vi "Martins HOT interface Mikrotron.vi"() -> ()   [LabVIEW 2012]
uses:
  Sub VIs/Trap cluster.ctl
  <vilib>/vision/Image Controls.llb/IMAQ Image.ctl
  Sub VIs/Get measurement coordinates.vi
  Sub VIs/Global variables.vi
  <vilib>/Utility/inputDevices.llb/closeKeyboard.vi
  <vilib>/Utility/inputDevices.llb/keyboardAcquire.vi
  <vilib>/Utility/file.llb/Write To Spreadsheet File (DBL).vi
  Sub VIs/Get trap pos.vi
  <vilib>/Analysis/coordinate.llb/2D Cartesian Coordinate Shift.vi
  <vilib>/Analysis/coordinate.llb/2D Cartesian Coordinate Shift (Array).vi
  <vilib>/Analysis/coordinate.llb/2D Cartesian Coordinate Rotation.vi
  <vilib>/Analysis/coordinate.llb/2D Cartesian Coordinate Rotation (Scalar).vi
  <vilib>/vision/driver/imaqhl.llb/IMAQ Grab Acquire.vi
  <vilib>/vision/driver/IMAQdx.llb/IMAQdx Grab.vi
  <vilib>/vision/driver/imaqll.llb/IMAQ Extract Buffer.vi
  <vilib>/vision/driver/NI_Vision_Acquisition_Software.lvlib
  <vilib>/vision/NI_Vision_Development_Module.lvlib
  <vilib>/Analysis/NI_AALPro.lvlib
panel:
  out "Using monitoring camera\nfor measurements":bool
  out "Measurement image":T1
  out "Monitoring image":T1
  in  "Apply Corrections":bool
  in  "View Licence":bool
  in  "ok":bool caption="Mark the center of \nthe spot using the \nzoom and the point\ntool, then click this \nbutton"
  in  "Stop program":bool
  in  "Updating trap cluster":bool=TRUE
  out "Camera enabled":bool=TRUE
  out "SLM enabled":bool=TRUE
  in  "Hologram generation":cluster{"Method":i32, "Iterations":i32}={"Method"=1, "Iterations"=30} {"Method" items=["Lenses & Gratings (3D)"=0, " Gerchberg-Saxton (3D)"=1, "Gerchberg-Saxton FFT (2D)"=2, "Nothing"=-1]}
  in  "ROI":T2={"Global Rectangle"=[970, 428, 1180, 694], "Contours"=[{"Contour Type"=0, "ROI Type"=1, "Points"=[970, 585]}, {"Contour Type"=0, "ROI Type"=1, "Points"=[1179, 693]}, {"Contour Type"=0, "ROI Type"=1, "Points"=[1117, 428]}]}
  out "Monitor image":T1(plugin-control)
  out "# recorded points":i32
  in  "Set\nBlacklevel":i32=155 min=50 max=200 step=1
  in  "Set \nFramerate":i32=1024
  in  "Calibration framerate":i32=4096
  in  "N samples":i32=512
  in  "Calibration \nruns":i32=100
  in  "Calibrate \ntraps":bool
  out "acquired FPS":dbl=4093.320235756385
  out "processed FPS":dbl=43.222003929273086
  in  "reset":bool
  out "threshold":sgl=76.0
  in  "Outer bound":dbl=10.0
  in  "Inner bound":dbl=-8.0
  in  "stop \nsqueezing":bool
  in  "Squeeze":bool
  in  "Run meas calibration":bool
  in  "Display hologram\nand computed \nimage plane":bool
  in  "Run calibration":bool
  in  "decrement":bool
  in  "Increment":bool
  in  "subtract\nbackground":bool=TRUE
  in  "store \nbackground":bool
  in  "Coordinate mapping \n(Monitor to Measurement)":T3={"cZ"=1.0, "cY"=0.41727, "cX"=-0.416, "sZ"=0.0, "sY"=-101.696, "sX"=595.2}
  in  "Transpose Measurement":bool
  out "Image\nsaturated":bool
  in  "Display meas image":bool=TRUE
  in  "Display ROIs":bool=TRUE
  out "Measurement image report":T4={"Mean Value"=0.18148804, "Standard Variation"=2.185048, "Minimal Value"=0.0, "Maximal Value"=43.0, "Area (calibrated)"=65536.0, "Area (pixels)"=65536, "%"=100.0, "Calibration Valid"=TRUE} {"Mean Value" format="%.2f"; "%" format="%.2f"; "Area (calibrated)" format="%.2f"; "Maximal Value" format="%.2f"; "Minimal Value" format="%.2f"; "Standard Variation" format="%.2f"}
  in  "Save image path":path=path "E:/David/SLM characterization/Measured data/120420 - Trapping" caption="start path"
  in  "save image":bool
  in  "Edit trap cluster":bool
  in  "Display data":bool=TRUE
  in  "Measure \nintensities":bool
  in  "Purge data":bool
  in  "ROI \nsize":dbl=26.0 min=2.0 step=2.0
  in  "Save data":bool
  in  "Record":bool
  in  "G":bool[](array[boolean])=[TRUE, TRUE, TRUE]
  out "Current trap pos":T5={"X (IMAQ)"=[819.0, 911.0, 1317.0], "Y (IMAQ)"=[426.0, 573.0, 653.0], "Z"=[0.0, 0.0, 0.0], "I"=[10.0, 10.0, 10.0], "Trap number"=[0, 1, 2], "ROI number"=[0, 1, 2], "Number of traps"=3, "Group"=[FALSE, FALSE, FALSE]}
  out "NI Vision error":errorcluster
  out "CUDA/SLM error":errorcluster
  in  "Cancel calibration":bool
  in  "Skip step if \ntimed out":bool
  in  "Display path":bool=TRUE
  out "Average step \ntime (ms)":dbl=15.483552631578947
  in  "Step \ntime \n(ms)":u32=100
  in  "Pause":bool
  in  "cancel path":bool
  out "Step \nskipped":bool
  in  "Path control":T6={"follow path"=FALSE, "Step \nlength"=0.1, "Arrive \nsimultaneously"=FALSE, "Synchronize traps"=FALSE, "Add current \npositions to path"=FALSE}
  in  "Create path":bool
  out "#":dbl[](array[numeric])=[0.0, 1.0, 2.0]
  in  "Group \nTraps":bool
  in  "Move \nHandle":bool
  in  "Coordinate mapping \n(IMAQ to SLM)":T3={"cZ"=1.0, "cY"=0.1530153, "cX"=0.15356821, "sZ"=-16.0, "sY"=-92.344734, "sX"=-118.0}
  in  "Transpose SLM":bool
  in  "I":dbl[](array[numeric])=[20.0, 20.0, 20.0]
  in  "Z":dbl[](array[numeric])=[0.0, 0.0, 0.0]
  # "Martin\nPersson 2011"
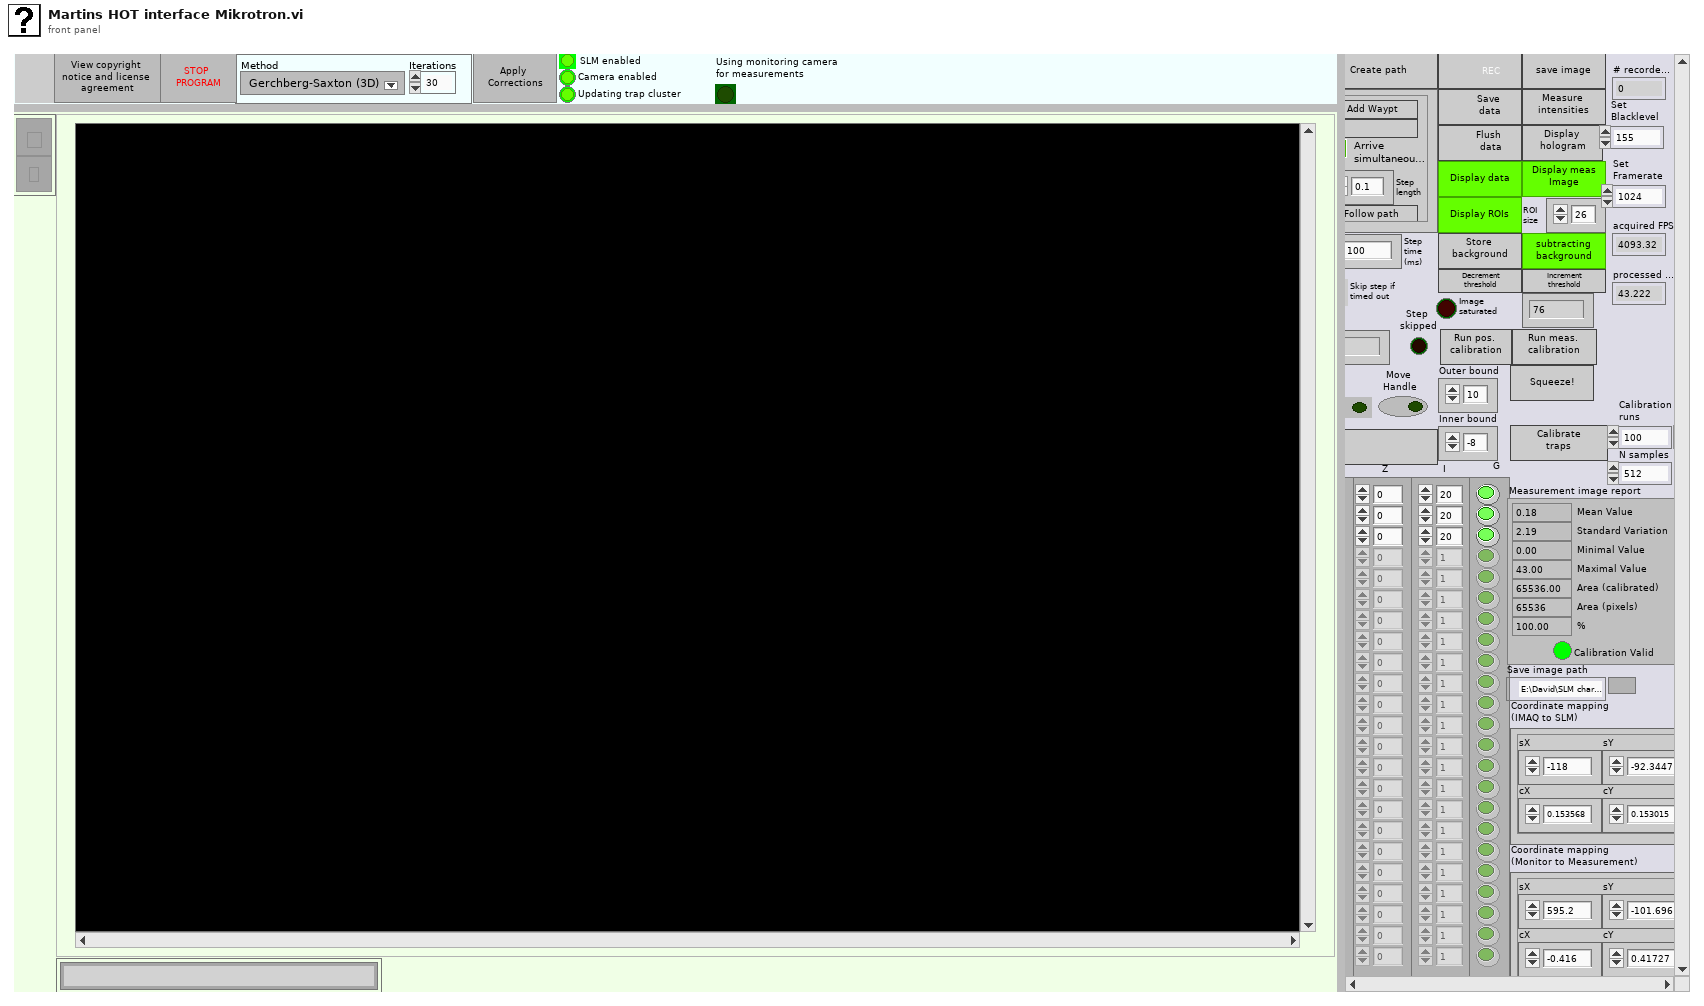
[diagram p1: front panel]
types:
  T1 = typedef "IMAQ Image.ctl" = refnum<image>
  T2 = cluster{"Global Rectangle":i32[], "Contours":cluster{"Contour Type":u32, "ROI Type":u32, "Points":i32[]}[]}
  T3 = cluster{"cZ":sgl, "cY":sgl, "cX":sgl, "sZ":sgl, "sY":sgl, "sX":sgl}
  T4 = cluster{"Mean Value":sgl, "Standard Variation":sgl, "Minimal Value":sgl, "Maximal Value":sgl, "Area (calibrated)":sgl, "Area (pixels)":u32, "%":sgl, "Calibration Valid":bool}
  T5 = typedef "Trap cluster.ctl" = cluster{"X (IMAQ)":sgl[], "Y (IMAQ)":sgl[], "Z":sgl[], "I":sgl[], "Trap number":i32[], "ROI number":i32[], "Number of traps":i32, "Group":bool[]}
  T6 = cluster{"follow path":bool, "Step \nlength":dbl, "Arrive \nsimultaneously":bool, "Synchronize traps":bool, "Add current \npositions to path":bool}
  T7 = cluster{"CentroidX":dbl[], "CentroidY":dbl[], "I":dbl[], "Acquired Buffer Number":u32}
  T8 = enum16{"IMAQ (Camera Link)", "IMAQ ring", "IMAQdx (firewire)", "No camera"}
  T9 = typedef "IMAQdx.ctl" = refnum<k21>
  T10 = cluster{"Camera type":enum16{"IMAQ (Camera Link)", "IMAQ ring", "IMAQdx (firewire)", "No camera"}, "IMAQ Session":refnum<k11>, "IMAQdx Session":T9, "Image":T1, "Image buffers":T1[], "Camera error":errorcluster}
  T11 = typedef "Image Type" = u32
  T12 = enum16{"0", "1", "2", "3", "4", "5", "6", "7", "8", "9", "A", "B", "C", "D", "E", "F", "G", "H", "I", "J", "K", "L", "M", "N", "O", "P", "Q", "R", "S", "T", "U", "V", "W", "X", "Y", "Z", "F1", "F2", "F3", "F4", "F5", "F6", "F7", "F8", "F9", "F10", "F11", "F12", "F13", "F14", "F15", "ADD", "BACK", "BACKSLASH", "CAPITAL", "COMMA", "DECIMAL", "DELETE", "DIVIDE", "DOWN", "END", "EQUALS", "ESCAPE", "GRAVE (`)", "HOME", "INSERT", "LBRACKET", "LCONTROL", "LEFT", "L ALT", "LSHIFT", "LWIN", "MINUS", "MULTIPLY", "NEXT", "NUMLOCK", "NUMPAD_0", "NUMPAD_1", "NUMPAD_2", "NUMPAD_3", "NUMPAD_4", "NUMPAD_5", "NUMPAD_6", "NUMPAD_7", "NUMPAD_8", "NUMPAD_9", "PAUSE", "PERIOD", "PRIOR (PG UP)", "RBRACKET", "RCONTROL", "RETURN", "RIGHT", "R ALT", "RSHIFT", "RWIN", "SCROLL", "SEMICOLON", "SLASH", "SPACE", "SUBTRACT", "TAB", "UP", "ENTER (num pad)", "' (quote)"}[]
  T13 = cluster{"CentroidX":dbl[], "CentroidY":dbl[], "I":dbl[], "Acquired Buffer Number":u32}[]
  T14 = enum16{"Left Button", "Center Button", "Right Button", "Window Close"}
  T15 = typedef "ROI Descriptor" = cluster{"Global Rectangle":i32[], "Contours":cluster{"ID":enum32{"External", "Internal"}, "Type":u32, "Coordinates":i32[]}[]}
  T16 = cluster{"Contour Type":u32, "ROI Type":u32, "Points":i32[]}[]
  T17 = cluster{"Contour Type":u32, "ROI Type":u32, "Points":i32[]}
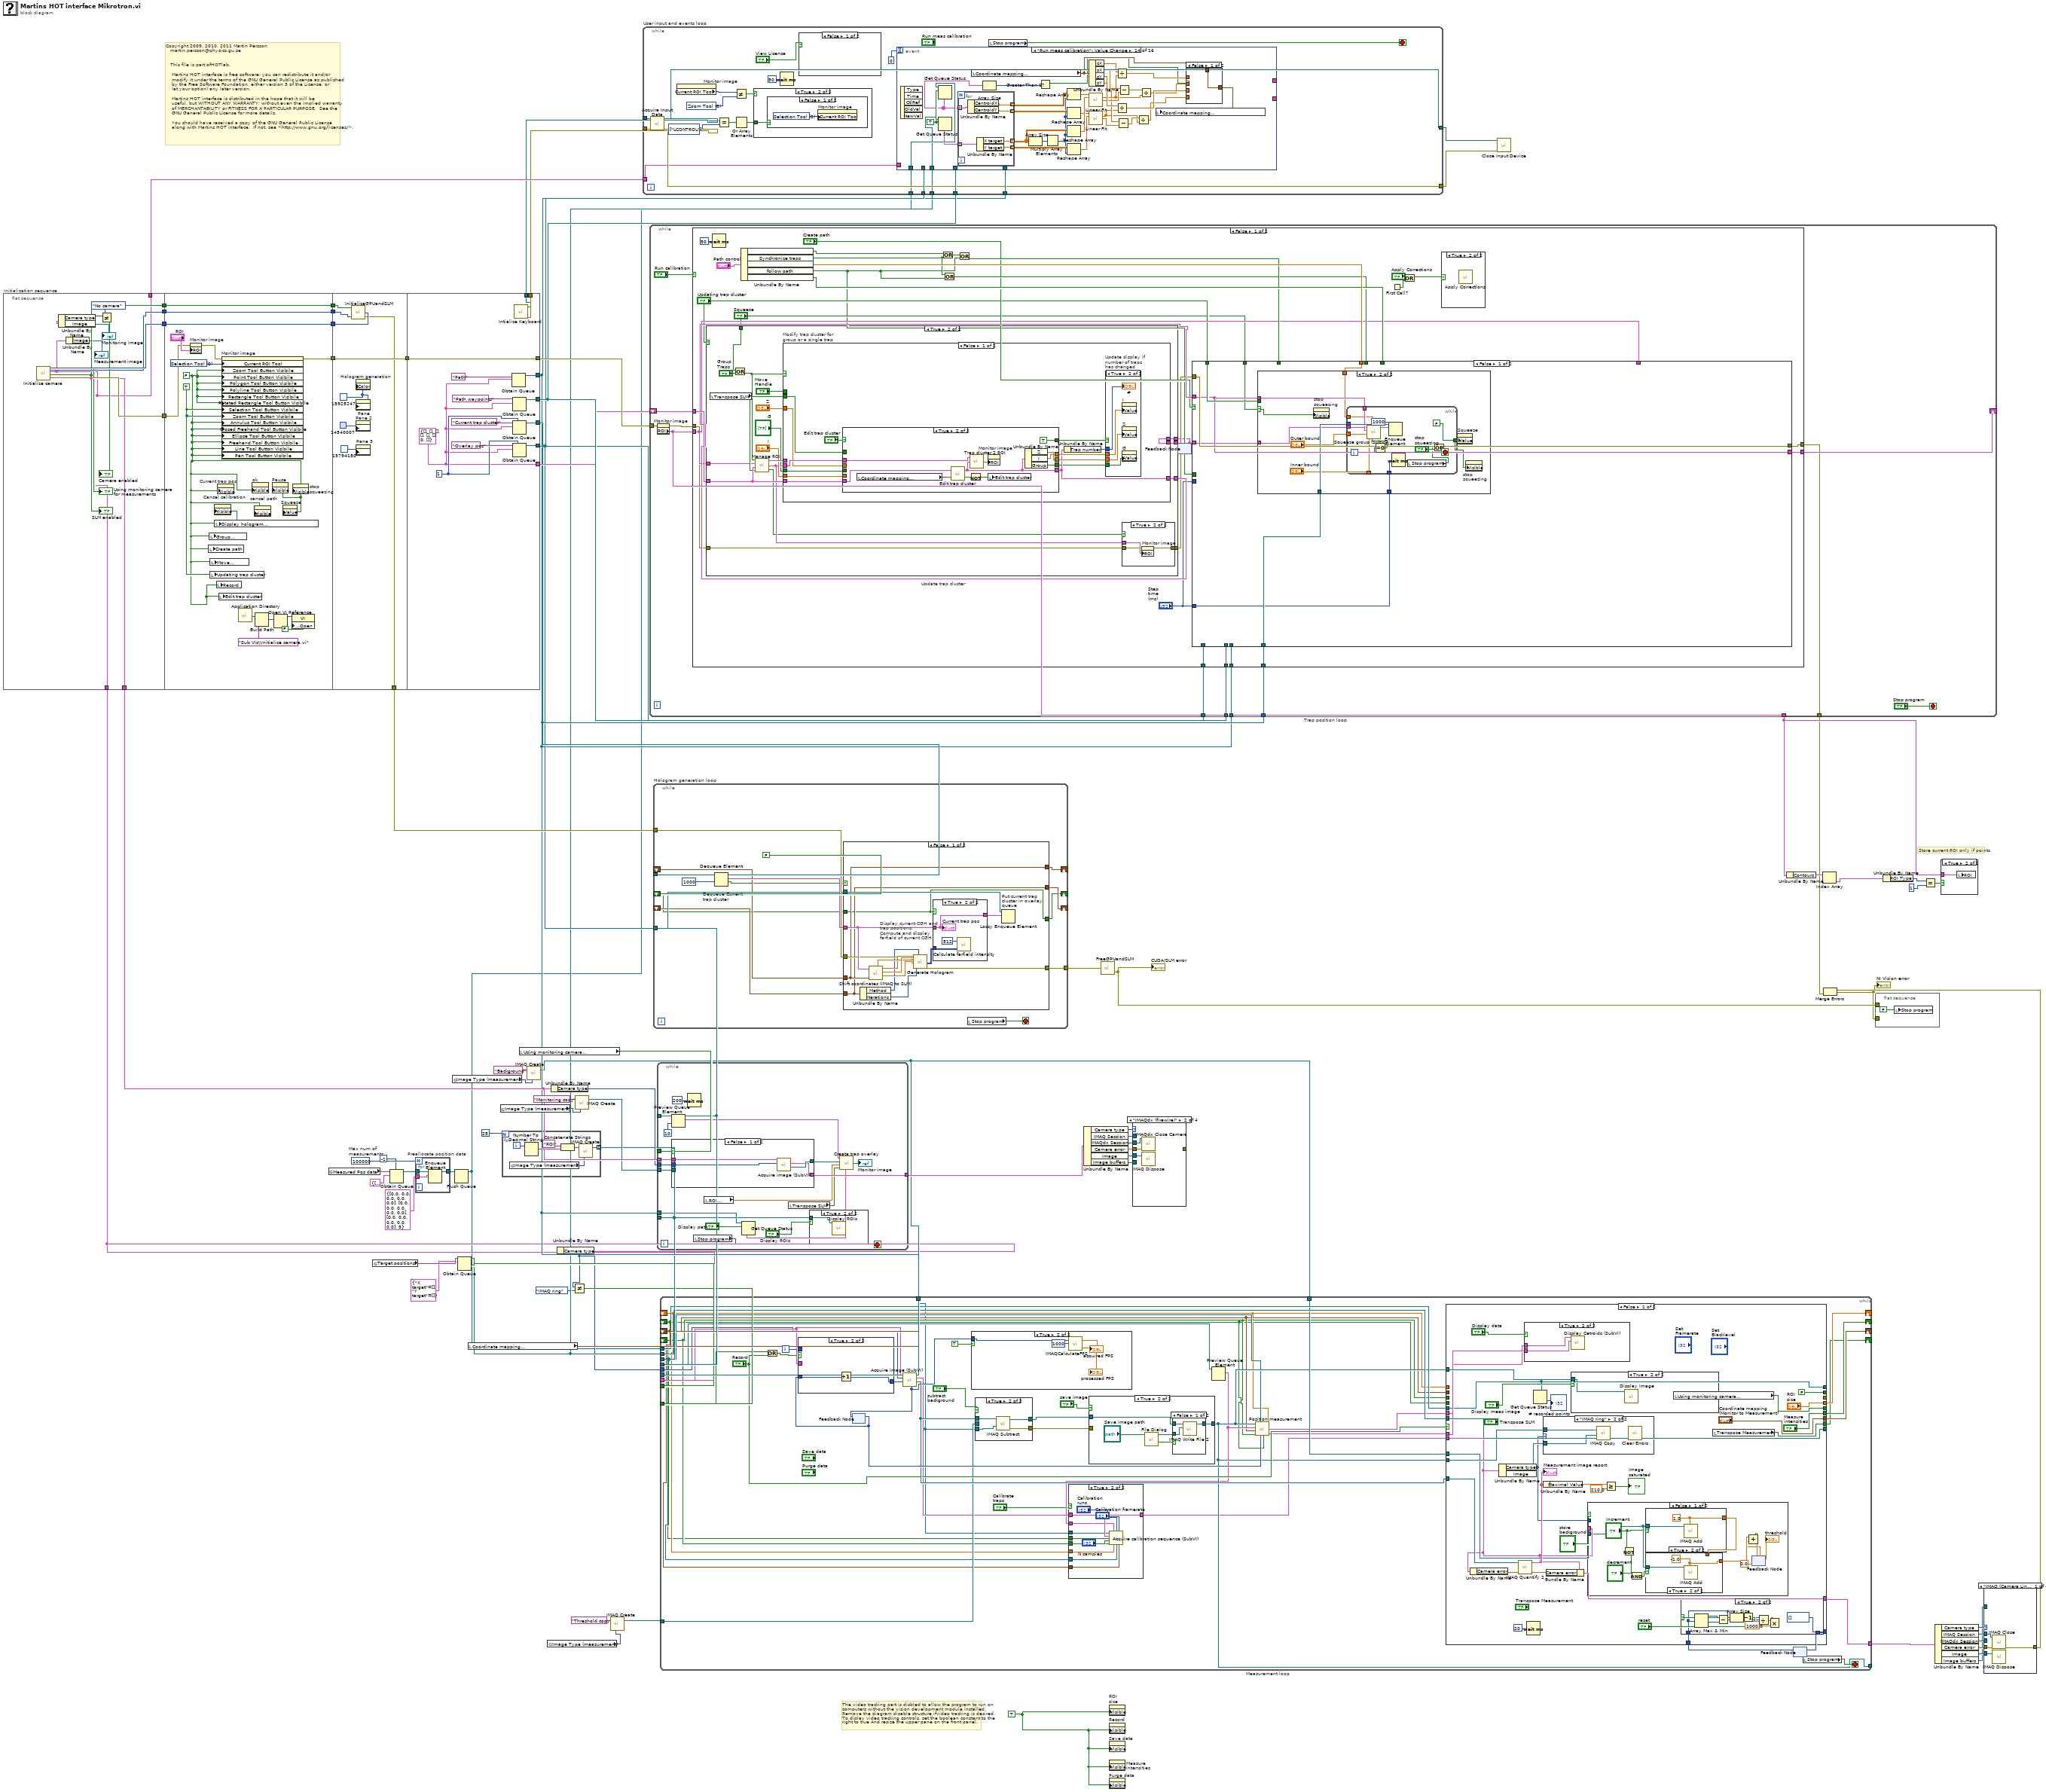
[diagram p0: block diagram]
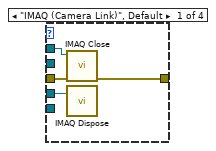
[diagram p2: hidden frame]
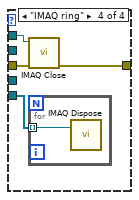
[diagram p4: hidden frame]
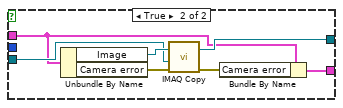
[diagram p6: hidden frame]
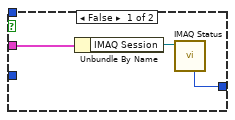
[diagram p10: hidden frame]
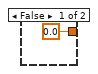
[diagram p17: hidden frame]
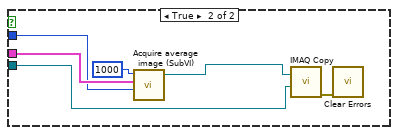
[diagram p18: hidden frame]
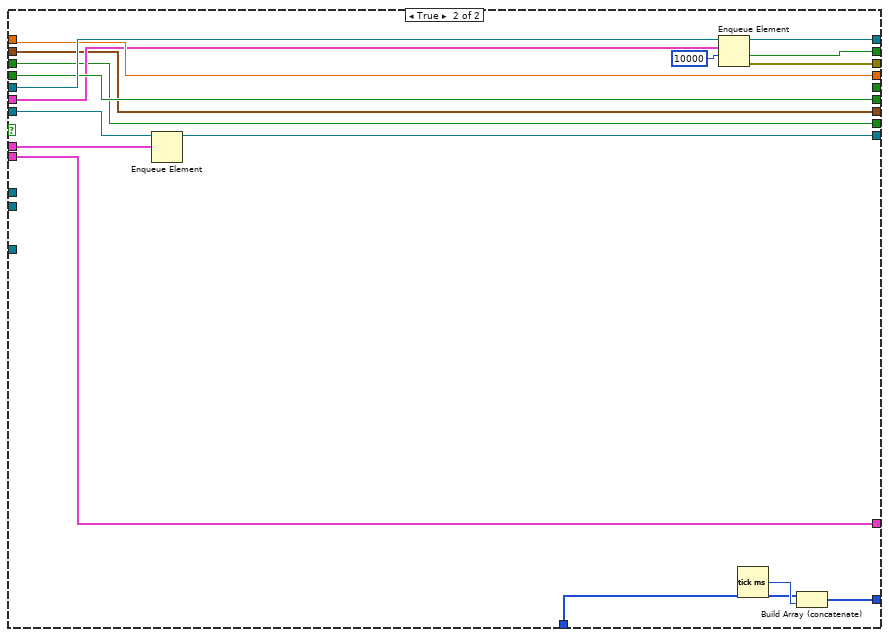
[diagram p20: hidden frame]
diagram:
  w11 = 100000  # Max num of  measurements
  w78 = TRUE ("Visible")
  # "Copyright 2009, 2010, 2011 Martin Persson \n   martin.persson@physics.gu.se\n\n\n   This file is part ofHOTlab.\n\n    Martins HOT interface is free software: you can redistribute it and/or \n    modify it under the terms of the GNU General Public License as published \n    by the Free Software Foundation, either version 3 of the License, or\n    (at your option) any later version.\n\n    Martins HOT interface is distributed in the hope that it will be \n    useful, but WITHOUT ANY WARRANTY; without even the implied warranty\n    of MERCHANTABILITY or FITNESS FOR A PARTICULAR PURPOSE.  See the\n    GNU General Public License for more details.\n\n    You should have received a copy of the GNU General Public License\n    along with Martins HOT interface.  If not, see <http://www.gnu.org/licenses/>."
  # "Store current ROI only if points"
  # "The video tracking part is disbled to allow the program to run on\ncomputers without the vision development module installed. \nRemove the diagram disable structure ifvideo tracking is desired. \nTo diplay video tracking controls, set the boolean constant to the \nright to true And resize the upper pane on the front panel."
  n1 = flat-sequence "Initialization sequence" {
    tunnel: [w88] -> w65
    tunnel: [w91] -> w64
    tunnel: [w90] -> w63
    tunnel: [w89] -> w62
    tunnel: [w83] -> w42
    tunnel: [w81] -> w15
    tunnel: [w81] -> w51
    tunnel: w65 -> [w104]
    tunnel: w64 -> [w102]
    tunnel: w63 -> [w106]
    tunnel: w62 -> [w105]
    tunnel: [w104] -> w58
    tunnel: [w99] -> w57
    tunnel: [w106] -> w55
    tunnel: [w105] -> w54
    tunnel: w58 -> [w111]
    tunnel: w57 -> [w114]
    tunnel: [w114] -> w56
    tunnel: w55 -> [w112]
    tunnel: w54 -> [w113]
    tunnel: [w110] -> w53
    tunnel: [w127] -> w61
    tunnel: w56 -> [w127]
    tunnel: [w125] -> w29
    tunnel: [w123] -> w60
    tunnel: [w121] -> w52
    tunnel: [w120] -> w30
    tunnel: [w117] -> w59
    tunnel: [w116] -> w2
    tunnel: [w115] -> w1
    frame #0 {
      n2 = call "Initialize camera.vi"() -> ("Use monitoring camera\nfor measurements"=→"Using monitoring camera\nfor measurements":bool, "Vision error out"=w91:errorcluster, "CUDA device ID"=w89:i32, "TrueFrame out"=w90:i32, "Measurement camera cluster"=w81:T10, "SLM enabled"=w88:bool, "Monitoring camera cluster"=w83:T10)  [unwired: 4 in]
      "SLM enabled" <- w88
      n3 = Unbundle By Name(w83) -> ("Camera type"=w85:T8, "Image"=→"Monitoring image":T1)
      n4 = Unbundle By Name(w81) -> ("Image"=→"Measurement image":T1)
      n5 = Not Equal?(x=w85, y=T8."No camera") -> (x != y?=→"Camera enabled":bool)
    }
    frame #1 {
      w98 = TRUE ("ROI Tool Buttons Visibile:Zoom Tool Button Visible")
      w97 = FALSE ("ROI Tool Buttons Visibile:Zoom Tool Button Visible")
      w101 = u32 0 items=["Zoom Tool"=8, "Selection Tool"=0, "Pan Tool"=9, "Point Tool"=1, "Line Tool"=2, "Rectangle Tool"=3, "Rotated Rectangle Tool"=12, "Polyline Tool"=10, "Polygon Tool"=5, "Freehand Tool"=11, "Closed Freehand Tool"=6, "Ellipse Tool"=4, "Annulus Tool"=7] ("Current ROI Tool")
      n6 = property on="Monitor image" class="ImageControl"(error in=w102, "ROI"="ROI") -> (error out=w100:errorcluster)  [unwired: 1 in, 1 out]
      n7 = local write "Create path"(w97) -> ()
      n8 = local write "Group \nTraps"(w97) -> ()
      n9 = local write "Move \nHandle"(w97) -> ()
      n10 = local write "Updating trap cluster"(w98) -> ()
      n11 = property on="Cancel calibration" class="Bool"("Visible"=w97) -> ()  [unwired: 2 in, 2 out]
      n12 = local write "Display hologram\nand computed \nimage plane"(w97) -> ()
      n13 = local write "Record"(w97) -> ()
      n14 = property on="Current trap pos" class="Clust (strict)"("Visible"=w97) -> ()  [unwired: 2 in, 2 out]
      n15 = local write "Edit trap cluster"(w97) -> ()
      n16 = property on="Monitor image" class="ImageControl"(error in=w100, "Current ROI Tool"=w101, "Zoom Tool Button Visibile"=w97, "Point Tool Button Visibile"=w97, "Polygon Tool Button Visibile"=w97, "Polyline Tool Button Visibile"=w97, "Rectangle Tool Button Visibile"=w97, "Rotated Rectangle Tool Button Visibile"=w97, "Selection Tool Button Visibile"=w98, "Zoom Tool Button Visibile"=w98, "Annulus Tool Button Visibile"=w97, "Closed Freehand Tool Button Visibile"=w97, "Ellipse Tool Button Visibile"=w97, "Freehand Tool Button Visibile"=w97, "Line Tool Button Visibile"=w97, "Pan Tool Button Visibile"=w97) -> (error out=w99:errorcluster)  [unwired: 1 in, 1 out]
      n17 = call <vilib>:"Application Directory.vi"() -> ("Application Directory"=w93:path)
      n18 = property on="ok" class="Bool"("Visible"=w97) -> ()  [unwired: 2 in, 2 out]
      n19 = property on="cancel path" class="Bool"("Visible"=w97) -> ()  [unwired: 2 in, 2 out]
      n20 = Build Path(base path=w93, name or relative path="Sub VIs\\Initialize camera.vi") -> (appended path=w96:path)
      n21 = property on="Pause" class="Bool (strict)"("Visible"=w97) -> ()  [unwired: 2 in, 2 out]
      n22 = Open VI Reference(vi path=w96) -> (vi reference=w95:refnum<vi>)  [unwired: 5 in, 1 out]
      n23 = property on="Squeeze" class="Bool (strict)"("Value"=w97) -> ()  [unwired: 2 in, 2 out]
      n24 = property class="VI"(reference=w95, "Front Panel.Open"=FALSE ("Front Panel Window:Open")) -> ()  [unwired: 1 in, 2 out]
      n25 = property on="stop \nsqueezing" class="Bool"("Visible"=w97) -> ()  [unwired: 2 in, 2 out]
    }
    frame #2 {
      w107 = u32 15925247 ("Pane Color")
      n26 = call "InitializeGPUandSLM.vi"("TrueFrame"=w112, "deviceId"=w113, "SLM enabled"=w111) -> ("CUDA/SLM error"=w110:errorcluster)  [unwired: 1 in, 1 out]
      n27 = property on="Hologram generation" class="Clust (strict)"("Color"=w107) -> ()  [unwired: 2 in, 2 out]
      n28 = property on="Pane" class="Pane"("PaneColor"=w107) -> ()  [unwired: 2 in, 2 out]
      n29 = property on="Pane 2" class="Pane"("PaneColor"=u32 14540007 ("Pane Color")) -> ()  [unwired: 2 in, 2 out]
      n30 = property on="Pane 3" class="Pane"("PaneColor"=u32 15794150 ("Pane Color")) -> ()  [unwired: 2 in, 2 out]
    }
    frame #3 {
      w117 = T5 {"X (IMAQ)"=[], "Y (IMAQ)"=[], "Z"=[], "I"=[], "Trap number"=[], "ROI number"=[], "Number of traps"=0, "Group"=[]} ("output cluster 2")
      w118 = 1 ("max queue size (-1, unlimited)")
      n31 = Obtain Queue(name (unnamed)="Path", element data type=w117) -> (queue out=w125:refnum<queue>)  [unwired: 3 in, 2 out]
      n32 = Obtain Queue(name (unnamed)="Path waypoints", element data type=w117) -> (queue out=w123:refnum<queue>)  [unwired: 3 in, 2 out]
      n33 = Obtain Queue(max queue size (-1, unlimited)=w118, name (unnamed)="Current trap cluster", element data type=w117) -> (queue out=w121:refnum<queue>)  [unwired: 2 in, 2 out]
      n34 = Obtain Queue(max queue size (-1, unlimited)=w118, name (unnamed)="Overlay pos", element data type=w117) -> (queue out=w120:refnum<queue>)  [unwired: 2 in, 2 out]
      n35 = call <vilib>:"Intialize Keyboard.vi"() -> ("error out"=w116:errorcluster, "device ID"=w115:refnum<k1>)  [unwired: 1 in, 9 out]
    }
  }
  n36 = global read "Global variables.vi" "Measured Pos data"() -> (w7:string)
  n37 = global read "Global variables.vi" "Target positions"() -> (w18:string)
  n38 = Obtain Queue(max queue size (-1, unlimited)=-1, name (unnamed)=w7, element data type=T7 {"CentroidX"=[], "CentroidY"=[], "I"=[], "Acquired Buffer Number"=0} ("Position data out")) -> (queue out=w8:refnum<queue>)  [unwired: 2 in, 2 out]
  n39 = for "Preallocate position data" {
    N: w11 -> [_]
    tunnel: w8 -> [w130]
    tunnel: T7 {"CentroidX"=[0.0, 0.0, 0.0, 0.0, 0.0], "CentroidY"=[0.0, 0.0, 0.0, 0.0, 0.0], "I"=[0.0, 0.0, 0.0, 0.0, 0.0], "Acquired Buffer Number"=5} ("Position data out") -> [w129]
    tunnel: [w128] -> w10
    n40 = Enqueue Element(queue=w130, element=w129) -> (queue out=w128:refnum<queue>)  [unwired: 2 in, 2 out]
  }
  n41 = global read "Global variables.vi" "Image Type (measurement)"() -> (w21:T11)
  n42 = Flush Queue(queue=w10) -> (queue out=w5:refnum<queue>)  [unwired: 1 in, 2 out]
  n43 = Obtain Queue(name (unnamed)=w18, element data type=cluster{"X target":sgl[], "Y target":sgl[]} {"X target"=[], "Y target"=[]} ("Target coordinates 2")) -> (queue out=w16:refnum<queue>, created new?=w17:bool)  [unwired: 3 in, 1 out]
  n44 = local read "Coordinate mapping \n(Monitor to Measurement)"() -> (w23:T3)
  n45 = global read "Global variables.vi" "Image Type (measurement)"() -> (w24:T11)
  n46 = for {
    N: 25 -> [_]
    tunnel: [w136] -> w28 mode=indexing
    i -> [w133]
    n47 = global read "Global variables.vi" "Image Type (measurement)"() -> (w131:T11)
    n48 = Number To Decimal String(number=w133) -> (decimal integer string=w132:string)  [unwired: 1 in]
    n49 = Concatenate Strings("ROI" ("Image Name"), w132) -> (w134:string)
    n50 = call "IMAQ Create"("Image Name"=w134, "Image Type"=w131) -> ("New Image"=w136:T1)  [unwired: 3 in, 1 out]
  }
  n51 = local read "Using monitoring camera\nfor measurements"() -> (w33:bool)
  n52 = call "IMAQ Create"("Image Name"="Background", "Image Type"=w21) -> ("New Image"=w19:T1)  [unwired: 3 in, 1 out]
  n53 = global read "Global variables.vi" "Image Type (measurement)"() -> (w25:T11)
  n54 = Unbundle By Name(w42) -> ("Camera type"=w34:T8)
  n55 = Unbundle By Name(w15) -> ("Camera type"=w13:T8)
  n56 = Not Equal?(x=w13, y=T8."IMAQ ring") -> (x != y?=w14:bool)
  n57 = call "IMAQ Create"("Image Name"="Monitoring copy", "Image Type"=w24) -> ("New Image"=w31:T1)  [unwired: 3 in, 1 out]
  n58 = call "IMAQ Create"("Image Name"="Threshold copy", "Image Type"=w25) -> ("New Image"=w27:T1)  [unwired: 3 in, 1 out]
  n59 = while "User input and events loop" {
    tunnel: w1 -> [w157]
    tunnel: w30 -> [w146]
    tunnel: w60 -> [w145]
    tunnel: w29 -> [w144]
    tunnel: [w143] -> w67
    tunnel: w2 -> [w142]
    tunnel: [w141] -> w66
    tunnel: w51 -> [w139]
    tunnel: w5 -> [w138]
    tunnel: w16 -> [w137]
    stop <- w149 stop-if-true
    w154 = u32 8 items=["Zoom Tool"=8, "Selection Tool"=0, "Pan Tool"=9, "Point Tool"=1, "Line Tool"=2, "Rectangle Tool"=3, "Rotated Rectangle Tool"=12, "Polyline Tool"=10, "Polygon Tool"=5, "Freehand Tool"=11, "Closed Freehand Tool"=6, "Ellipse Tool"=4, "Annulus Tool"=7] ("Current ROI Tool")
    w151 = T12 [enum."LCONTROL"] items=["0", "1", "2", "3", "4", "5", "6", "7", "8", "9", "A", "B", "C", "D", "E", "F", "G", "H", "I", "J", "K", "L", "M", "N", "O", "P", "Q", "R", "S", "T", "U", "V", "W", "X", "Y", "Z", "F1", "F2", "F3", "F4", "F5", "F6", "F7", "F8", "F9", "F10", "F11", "F12", "F13", "F14", "F15", "ADD", "BACK", "BACKSLASH", "CAPITAL", "COMMA", "DECIMAL", "DELETE", "DIVIDE", "DOWN", "END", "EQUALS", "ESCAPE", "GRAVE (`)", "HOME", "INSERT", "LBRACKET", "LCONTROL", "LEFT", "L ALT", "LSHIFT", "LWIN", "MINUS", "MULTIPLY", "NEXT", "NUMLOCK", "NUMPAD_0", "NUMPAD_1", "NUMPAD_2", "NUMPAD_3", "NUMPAD_4", "NUMPAD_5", "NUMPAD_6", "NUMPAD_7", "NUMPAD_8", "NUMPAD_9", "PAUSE", "PERIOD", "PRIOR (PG UP)", "RBRACKET", "RCONTROL", "RETURN", "RIGHT", "R ALT", "RSHIFT", "RWIN", "SCROLL", "SEMICOLON", "SLASH", "SPACE", "SUBTRACT", "TAB", "UP", "ENTER (num pad)", "' (quote)"] ("keys pressed")
    n60 = call-poly <vilib>:"Acquire Input Data.vi"("device ID"=w157, "error in (no error)"=w142) -> ("device ID"=w143:refnum<k1>, "keys pressed"=w150:T12, "error out"=w141:errorcluster)  [unwired: 15 out]
    n61 = property on="Monitor image" class="ImageControl"() -> ("Current ROI Tool"=w153:u32)  [unwired: 2 in, 2 out]
    n62 = Equal?(x=w150, y=w151) -> (x = y?=w152:bool[])
    n63 = Not Equal?(x=w153, y=w154) -> (x != y?=w155:bool)
    n64 = Or Array Elements(Boolean array=w152) -> (logical OR=w156:bool)
    n65 = case shown="True" w155 {
      tunnel: w156 -> [_ w277]
      frame False {
      }
      frame True {
        n66 = case shown="False" w277 {
          frame False {
            w278 = u32 0 items=["Zoom Tool"=8, "Selection Tool"=0, "Pan Tool"=9, "Point Tool"=1, "Line Tool"=2, "Rectangle Tool"=3, "Rotated Rectangle Tool"=12, "Polyline Tool"=10, "Polygon Tool"=5, "Freehand Tool"=11, "Closed Freehand Tool"=6, "Ellipse Tool"=4, "Annulus Tool"=7] ("Current ROI Tool")
            n67 = property on="Monitor image" class="ImageControl"("Current ROI Tool"=w278) -> ()  [unwired: 2 in, 2 out]
          }
          frame True {
            w279 = u32 1 items=["Zoom Tool"=8, "Selection Tool"=0, "Pan Tool"=9, "Point Tool"=1, "Line Tool"=2, "Rectangle Tool"=3, "Rotated Rectangle Tool"=12, "Polyline Tool"=10, "Polygon Tool"=5, "Freehand Tool"=11, "Closed Freehand Tool"=6, "Ellipse Tool"=4, "Annulus Tool"=7] ("Current ROI Tool")
            n68 = property on="Monitor image" class="ImageControl"("Current ROI Tool"=w279) -> ()  [unwired: 2 in, 2 out]
          }
        }
      }
    }
    n69 = Wait (ms)(milliseconds to wait=u32 50) -> ()  [unwired: 1 out]
    n70 = case shown="False" "View Licence" {
      frame False {
      }
      frame True {
        n71 = call "View license.vi"() -> ()  [unwired: 1 in]
      }
    }
    n72 = event shown="[13] \"Run meas calibration\": Value Change" {
      selector: _ -> [_ _ _ _ _ _ _ _ _ _ _ _ _ _ _ _]
      dyn-events: _ -> [_ _ _ _ _ _ _ _ _ _ _ _ _ _ _ _]
      timeout: 0 -> [_ _ _ _ _ _ _ _ _ _ _ _ _ _ _ _]
      tunnel: w146 -> [_ _ w164 _ _ _ _ _ _ _ _ _ _ _ _ _]
      tunnel: w145 -> [_ _ w163 _ _ _ _ _ _ _ _ _ _ _ _ _]
      tunnel: w144 -> [_ _ w167 _ _ _ _ _ _ _ _ _ _ _ _ _]
      tunnel: w139 -> [_ _ _ _ _ _ w180 _ _ _ _ _ _ _ w273 w276]
      tunnel: w138 -> [_ _ _ _ _ _ _ _ _ _ _ w200 w224 w257 _ _]
      tunnel: w137 -> [_ _ _ _ _ _ _ _ _ _ _ w199 w223 w256 _ _]
      tunnel: [_ _ _ _ _ _ _ _ _ _ _ _ w222 _ _ _] -> _
      tunnel: [_ _ _ _ _ _ _ _ _ _ _ _ w221 _ _ _] -> _
      event Timeout {
        n73 = event-data() -> ()  [unwired: 1 in, 2 out]
      }
      event "Display hologram\nand computed \nimage plane": Value Change {
        n74 = event-data() -> ("NewVal"=w158:bool)  [unwired: 1 in, 4 out]
        n75 = property on="Current trap pos" class="Clust (strict)"("Visible"=w158) -> ()  [unwired: 2 in, 2 out]
        n76 = call <vilib>:"Application Directory.vi"() -> ("Application Directory"=w159:path)
        n77 = Build Path(base path=w159, name or relative path="Sub VIs\\Calculate farfield intensity.vi") -> (appended path=w162:path)
        n78 = Open VI Reference(vi path=w162) -> (vi reference=w161:refnum<vi>)  [unwired: 5 in, 1 out]
        n79 = property class="VI"(reference=w161, "Front Panel.Open"=w158) -> ()  [unwired: 1 in, 2 out]
      }
      event "Create path": Value Change {
        n80 = event-data() -> ()  [unwired: 1 in, 5 out]
        n81 = property on="follow path" class="Bool (strict)"("Value"=FALSE) -> ()  [unwired: 2 in, 2 out]
        n82 = Flush Queue "Flush path \nwaypt queue"(queue=w163) -> ()  [unwired: 1 in, 3 out]
        n83 = Preview Queue Element(queue=w164) -> (element=w165:T5, error out=w168:errorcluster)  [unwired: 2 in, 2 out]
        n84 = Flush Queue "Flush path queue"(queue=w167) -> (queue out=w166:refnum<queue>)  [unwired: 1 in, 2 out]
        n85 = Enqueue Element "Enqueue current \ntrap pos in path"(queue=w166, element=w165) -> ()  [unwired: 2 in, 3 out]
        n86 = Enqueue Element "Enqueue current \ntrap pos in path \nwaypts"(queue=w163, element=w165, error in (no error)=w168) -> ()  [unwired: 1 in, 3 out]
      }
      event "cancel path": Value Change {
        n87 = event-data() -> ()  [unwired: 1 in, 5 out]
        n88 = local write "Create path"(FALSE ("Visible")) -> ()
      }
      event "Monitor image", "Group \nTraps", "Z", "I", "Coordinate mapping \n(IMAQ to SLM)": Mouse Down {
        w171 = FALSE ("Edit trap cluster")
        n89 = event-data() -> ()  [unwired: 1 in, 7 out]
        n90 = local write "Updating trap cluster"(TRUE ("Update trap positions")) -> ()
        n91 = local write "Edit trap cluster"(w171) -> ()
        n92 = call <vilib>:"Application Directory.vi"() -> ("Application Directory"=w172:path)
        n93 = Build Path(base path=w172, name or relative path="Sub VIs\\Edit trap cluster.vi") -> (appended path=w175:path)
        n94 = Open VI Reference(vi path=w175) -> (vi reference=w174:refnum<vi>)  [unwired: 5 in, 1 out]
        n95 = property class="VI"(reference=w174, "Front Panel.Open"=w171) -> ()  [unwired: 1 in, 2 out]
      }
      event "Group \nTraps", "Z", "I", "Monitor image", "Coordinate mapping \n(IMAQ to SLM)": Mouse Up {
        n96 = event-data() -> ()  [unwired: 1 in, 7 out]
        n97 = flat-sequence {
          frame #0 {
            n98 = Wait (ms)(milliseconds to wait=u32 100) -> ()  [unwired: 1 out]
          }
          frame #1 {
            n99 = local write "Updating trap cluster"(FALSE ("Update trap positions")) -> ()
          }
        }
      }
      event "Record": Value Change {
        n100 = event-data() -> ()  [unwired: 1 in, 5 out]
        n101 = Unbundle By Name(w180) -> ("Image buffers"=w179:T1[])
        n102 = for {
          tunnel: w179 -> [w181] mode=indexing
          n103 = call "IMAQ Clear Overlay"("Image"=w181) -> ()  [unwired: 9 in, 2 out]
        }
      }
      event "Display data": Value Change {
        n104 = event-data() -> ("NewVal"=w183:bool)  [unwired: 1 in, 4 out]
        n105 = call <vilib>:"Application Directory.vi"() -> ("Application Directory"=w182:path)
        n106 = Build Path(base path=w182, name or relative path="Sub VIs\\Display Cetroids (SubVI).vi") -> (appended path=w186:path)
        n107 = Open VI Reference(vi path=w186) -> (vi reference=w185:refnum<vi>)  [unwired: 5 in, 1 out]
        n108 = property class="VI"(reference=w185, "Front Panel.Open"=w183) -> ()  [unwired: 1 in, 2 out]
      }
      event "Display ROIs": Value Change {
        n109 = event-data() -> ("NewVal"=w187:bool)  [unwired: 1 in, 4 out]
        n110 = call <vilib>:"Application Directory.vi"() -> ("Application Directory"=w188:path)
        n111 = Build Path(base path=w188, name or relative path="Sub VIs\\Display ROIs.vi") -> (appended path=w191:path)
        n112 = Open VI Reference(vi path=w191) -> (vi reference=w190:refnum<vi>)  [unwired: 5 in, 1 out]
        n113 = property class="VI"(reference=w190, "Front Panel.Open"=w187) -> ()  [unwired: 1 in, 2 out]
      }
      event "Display meas image": Value Change {
        n114 = event-data() -> ("NewVal"=w192:bool)  [unwired: 1 in, 4 out]
        n115 = call <vilib>:"Application Directory.vi"() -> ("Application Directory"=w193:path)
        n116 = Build Path(base path=w193, name or relative path="Sub VIs\\Display Image.vi") -> (appended path=w196:path)
        n117 = Open VI Reference(vi path=w196) -> (vi reference=w195:refnum<vi>)  [unwired: 5 in, 1 out]
        n118 = property class="VI"(reference=w195, "Front Panel.Open"=w192) -> ()  [unwired: 1 in, 2 out]
      }
      event "Edit trap cluster": Value Change {
        n119 = event-data() -> ("NewVal"=w197:bool)  [unwired: 1 in, 4 out]
        n120 = local write "Updating trap cluster"(w197) -> ()
      }
      event "Save data": Value Change {
        n121 = event-data() -> ()  [unwired: 1 in, 5 out]
        n122 = Flush Queue(queue=w200) -> (remaining elements=w210:T13)  [unwired: 1 in, 2 out]
        n123 = Flush Queue(queue=w199) -> (remaining elements=w205:cluster{"X target":sgl[], "Y target":sgl[]}[])  [unwired: 1 in, 2 out]
        n124 = for {
          tunnel: [w220] -> w213 mode=indexing
          tunnel: [w219] -> w212 mode=indexing
          tunnel: [w218] -> w206 mode=indexing
          tunnel: w210 -> [w217] mode=indexing
          tunnel: w205 -> [w216] mode=indexing
          tunnel: [w215] -> w204 mode=indexing
          tunnel: [w214] -> w203 mode=indexing
          n125 = Unbundle By Name(w217) -> ("CentroidX"=w220:dbl[], "CentroidY"=w219:dbl[], "Acquired Buffer Number"=w218:u32)
          n126 = Unbundle By Name(w216) -> ("X target"=w215:sgl[], "Y target"=w214:sgl[])
        }
        n127 = Transpose 2D Array(2D array=w213) -> (transposed array=w209:dbl[][])
        n128 = Transpose 2D Array(2D array=w212) -> (transposed array=w208:dbl[][])
        n129 = Transpose 2D Array(2D array=w204) -> (transposed array=w202:sgl[][])
        n130 = Transpose 2D Array(2D array=w203) -> (transposed array=w201:sgl[][])
        n131 = Build Array (concatenate)(w206, w209, w208, w202, w201) -> (w198:dbl[][])
        n132 = Transpose 2D Array(2D array=w198) -> (transposed array=w207:dbl[][])
        n133 = call-poly <vilib>:"Write To Spreadsheet File.vi"("format (%.3f)"="%.9f", "2D data"=w207) -> ()  [unwired: 6 in, 1 out]
      }
      event "Purge data": Value Change {
        n134 = event-data() -> ()  [unwired: 1 in, 5 out]
        n135 = Flush Queue(queue=w224) -> (remaining elements=w222:T13)  [unwired: 1 in, 2 out]
        n136 = Flush Queue(queue=w223) -> (remaining elements=w221:cluster{"X target":sgl[], "Y target":sgl[]}[])  [unwired: 1 in, 2 out]
      }
      event "Run meas calibration": Value Change {
        w255 = TRUE ("return elements? (F)")
        n137 = event-data() -> ()  [unwired: 1 in, 5 out]
        n138 = Get Queue Status(queue=w257, return elements? (F)=w255) -> (elements=w227:T13)  [unwired: 1 in, 7 out]
        n139 = Get Queue Status(queue=w256, return elements? (F)=w255) -> (elements=w254:cluster{"X target":sgl[], "Y target":sgl[]}[])  [unwired: 1 in, 7 out]
        n140 = for {
          tunnel: w227 -> [w270] mode=indexing
          tunnel: w254 -> [w269] mode=indexing
          tunnel: [w268] -> w249 mode=indexing
          tunnel: [w267] -> w251 mode=indexing
          tunnel: [w266] -> w248 mode=indexing
          tunnel: [w265] -> w246 mode=indexing
          n141 = Unbundle By Name(w270) -> ("CentroidX"=w267:dbl[], "CentroidY"=w266:dbl[])
          n142 = Unbundle By Name(w269) -> ("X target"=w268:sgl[], "Y target"=w265:sgl[])
        }
        n143 = local read "Coordinate mapping \n(Monitor to Measurement)"() -> (w242:T3)
        n144 = Array Size(array=w227) -> (size(s)=w226:i32)
        n145 = Array Size(array=w249) -> (size(s)=w252:i32[])
        n146 = Greater Than 0?(x=w226) -> (x > 0?=w225:bool)
        n147 = Multiply Array Elements(1:w252) -> (0:w243:i32)
        n148 = Reshape Array(w251, w243) -> (w250:dbl[])
        n149 = Reshape Array(w248, w243) -> (w247:dbl[])
        n150 = Reshape Array(w249, w243) -> (w253:sgl[])
        n151 = Reshape Array(w246, w243) -> (w245:sgl[])
        n152 = Unbundle By Name(w242) -> ("cX"=w241:sgl, "sX"=w238:sgl, "cY"=w240:sgl, "sY"=w232:sgl)
        n153 = call <vilib>:"Linear Fit.vi"("Y"=w250, "X"=w253) -> ("slope"=w234:dbl, "intercept"=w237:dbl)  [unwired: 9 in, 3 out]
        n154 = call <vilib>:"Linear Fit.vi"("Y"=w247, "X"=w245) -> ("slope"=w229:dbl, "intercept"=w231:dbl)  [unwired: 9 in, 3 out]
        n155 = Divide(x=w241, y=w234) -> (x/y=w239:dbl)
        n156 = Divide(x=w240, y=w229) -> (x/y=w236:dbl)
        n157 = Subtract(x=w232, y=w231) -> (x-y=w230:dbl)
        n158 = Subtract(x=w238, y=w237) -> (x-y=w235:dbl)
        n159 = Divide(x=w230, y=w229) -> (x/y=w228:dbl)
        n160 = Divide(x=w235, y=w234) -> (x/y=w233:dbl)
        n161 = case shown="False" w225 {
          tunnel: [w258 w264] -> w244
          tunnel: w242 -> [w258 w263]
          tunnel: w239 -> [_ w262]
          tunnel: w236 -> [_ w261]
          tunnel: w233 -> [_ w260]
          tunnel: w228 -> [_ w259]
          frame False {
          }
          frame True {
            n162 = Bundle By Name(cluster=w263, "cX"=w262, "sX"=w260, "cY"=w261, "sY"=w259) -> (w264:T3)
          }
        }
        n163 = local write "Coordinate mapping \n(Monitor to Measurement)"(w244) -> ()
      }
      event "Set \nFramerate": Value Change {
        n164 = event-data() -> ("NewVal"=w271:i32)  [unwired: 1 in, 4 out]
        n165 = Unbundle By Name(w273) -> ("IMAQ Session"=w272:refnum<k11>)
        n166 = call "Set framerate (SubVI).vi"("Framerate"=w271, "IMAQ Refnum in"=w272) -> ()  [unwired: 7 in, 3 out]
      }
      event "Set\nBlacklevel": Value Change {
        n167 = event-data() -> ("NewVal"=w274:i32)  [unwired: 1 in, 4 out]
        n168 = Unbundle By Name(w276) -> ("IMAQ Session"=w275:refnum<k11>)
        n169 = call "Set blacklevel (SubVI).vi"("Blacklevel"=w274, "IMAQ Refnum in"=w275) -> ()  [unwired: 8 in, 2 out]
      }
    }
    n170 = local read "Stop program"() -> (w149:bool)
  }
  n171 = while "Trap position loop" {
    tunnel: w60 -> [w291]
    tunnel: w29 -> [w288]
    shift-right: [w290] -> _
    shift-left: w59 -> [w283]
    tunnel: w52 -> [w289]
    tunnel: w30 -> [w286]
    tunnel: [w285] -> w72
    tunnel: w61 -> [w282]
    tunnel: [w280] -> w70
    stop <- "Stop program" stop-if-true
    n172 = property on="Monitor image" class="ImageControl"(error in=w282) -> (error out=w281:errorcluster, "ROI"=w285:T2)  [unwired: 1 in, 1 out]
    n173 = case shown="False" "Run calibration" {
      selector: "Run calibration" -> [_ w539]
      tunnel: w291 -> [w321 _]
      tunnel: w283 -> [w320 w538]
      tunnel: [w300 w538] -> w290
      tunnel: w289 -> [w310 w547]
      tunnel: w288 -> [w309 _]
      tunnel: w286 -> [w306 _]
      tunnel: w285 -> [w305 w546]
      tunnel: w281 -> [w304 w543]
      tunnel: [w302 w540] -> w280
      frame False {
        n174 = Wait (ms)(milliseconds to wait=u32 50) -> ()  [unwired: 1 out]
        n175 = Unbundle By Name("Path control") -> ("Add current \npositions to path"=w307:bool, "Synchronize traps"=w315:bool, "Step \nlength"=w318:dbl, "follow path"=w294:bool, "Arrive \nsimultaneously"=w317:bool)
        n176 = Or(x=w307, y=w315) -> (x .or. y?=w316:bool)
        n177 = Or(x=w315, y=w294) -> (x .or. y?=w313:bool)
        n178 = Or(x=w316, y=w294) -> (x .or. y?=w314:bool)
        n179 = feedback #1() -> (w292:T2)  [unwired: 1 in]
        n180 = case "Update trap cluster" shown="True" "Updating trap cluster" {
          tunnel: w320 -> [w324 w342]
          tunnel: [w324 w335] -> w311
          tunnel: w305 -> [_ w333]
          tunnel: w304 -> [w323 w332]
          tunnel: [w323 w331] -> w303
          tunnel: "Squeeze" -> [_ w327]
          tunnel: [w322 w326] -> w293
          tunnel: w292 -> [w322 w325]
          frame False {
          }
          frame True {
            n181 = local read "Transpose SLM"() -> (w341:bool)
            n182 = Or(x=w327, y="Group \nTraps") -> (x .or. y?=w328:bool)
            n183 = call "Manage ROI.vi"("Switch X/Y"=w341, "Trap cluster in"=w342, "ROI in"=w333, "Group traps"=w328) -> ("Replace ROI"=w329:bool, "ROI out"=w334:T2, "Previous ROI out"=w340:T2)
            n184 = case "Modify trap cluster for \ngroup or a single trap" shown="False" w328 {
              tunnel: [w353 w393] -> w335
              tunnel: w334 -> [w360 w387]
              tunnel: w342 -> [w359 w395]
              tunnel: w340 -> [_ w394]
              tunnel: "Z" -> [w358 w392]
              tunnel: "Move \nHandle" -> [_ w391]
              tunnel: w341 -> [w357 w390]
              tunnel: "I" -> [w355 w389]
              tunnel: "G" -> [w350 w388]
              tunnel: [w347 w387] -> w326
              tunnel: w325 -> [w347 _]
              frame False {
                n185 = case shown="True" "Edit trap cluster" {
                  tunnel: w360 -> [w371 w374]
                  tunnel: w359 -> [w370 w382]
                  tunnel: w358 -> [w369 _]
                  tunnel: w357 -> [w368 _]
                  tunnel: [w367 w381] -> w356
                  tunnel: w355 -> [w366 _]
                  tunnel: [w365 w380] -> w354
                  tunnel: [w364 w376] -> w353
                  tunnel: [w363 TRUE ("Update display")] -> w351
                  tunnel: w350 -> [w362 _]
                  tunnel: [w361 w378] -> w349
                  frame False {
                    n186 = call "ROI 2 Trap Cluster.vi"("Amplitudes"=w366, "Switch X/Y"=w368, "Group"=w362, "Trap Cluster in"=w370, "Z"=w369, "ROI"=w371) -> ("Group out"=w361:bool[], "Z out"=w367:dbl[], "Amplitudes out"=w365:dbl[], "Trap Cluster Out"=w364:T5, "Update display"=w363:bool)
                  }
                  frame True {
                    n187 = local read "Coordinate mapping \n(IMAQ to SLM)"() -> (w373:T3)
                    n188 = call "Edit trap cluster.vi"("Coordinate mapping \n(IMAQ to SLM)"=w373, "trap cluster in"=w382) -> ("SubVI closed"=w377:bool, "Trap cluster out"=w376:T5)
                    n189 = Not(x=w377) -> (.not. x?=w372:bool)
                    n190 = call "Trap cluster 2 ROI.vi"("Trap cluster"=w376, "ROI in"=w374) -> ("ROI out"=w375:T2)  [unwired: 1 in]
                    n191 = property on="Monitor image" class="ImageControl"("ROI"=w375) -> ()  [unwired: 2 in, 2 out]
                    n192 = local write "Edit trap cluster"(w372) -> ()
                    n193 = Unbundle By Name(w376) -> ("Z"=w381:sgl[], "I"=w380:sgl[], "Group"=w378:bool[])
                  }
                }
                n194 = Unbundle By Name(w353) -> ("Trap number"=w352:i32[])
                n195 = case "Update display if\nnumber of traps \nhas changed" shown="True" w351 {
                  tunnel: w356 -> [_ w386]
                  tunnel: w354 -> [_ w385]
                  tunnel: w352 -> [_ w384]
                  tunnel: w349 -> [_ w383]
                  frame False {
                  }
                  frame True {
                    n196 = property on="I" class="Arr (strict)"("Value"=w385) -> ()  [unwired: 2 in, 2 out]
                    n197 = property on="Z" class="Arr (strict)"("Value"=w386) -> ()  [unwired: 2 in, 2 out]
                    n198 = property on="G" class="Arr (strict)"("Value"=w383) -> ()  [unwired: 2 in, 2 out]
                    "#" <- w384
                  }
                }
              }
              frame True {
                n199 = call "Move group.vi"("New handle position in"=w387, "Trap cluster in"=w395, "Previous handle position in"=w394, "Amplitudes"=w389, "Group"=w388, "Switch X/Y"=w390, "Move handle"=w391, "Z"=w392) -> ("Trap cluster out"=w393:T5)
              }
            }
            n200 = case shown="True" w329 {
              tunnel: w334 -> [_ w346]
              tunnel: w332 -> [w343 w345]
              tunnel: [w343 w344] -> w331
              frame False {
              }
              frame True {
                n201 = property on="Monitor image" class="ImageControl"(error in=w345, "ROI"=w346) -> (error out=w344:errorcluster)  [unwired: 1 in, 1 out]
              }
            }
          }
        }
        n202 = feedback-in #1(w293) -> ()
        n203 = case shown="False" "Create path" {
          tunnel: w321 -> [_ w440]
          tunnel: w311 -> [w400 w434]
          tunnel: w318 -> [w396 w449]
          tunnel: w309 -> [_ w444]
          tunnel: w317 -> [_ w448]
          tunnel: w314 -> [_ w447]
          tunnel: w313 -> [_ w446]
          tunnel: w294 -> [_ w445]
          tunnel: w310 -> [w403 w441]
          tunnel: w306 -> [_ w439]
          tunnel: w305 -> [_ w438]
          tunnel: w303 -> [w402 w437]
          tunnel: [w402 w436] -> w302
          tunnel: "Updating trap cluster" -> [w401 _]
          tunnel: [w400 w435] -> w300
          tunnel: "Squeeze" -> [w399 _]
          tunnel: w292 -> [w398 _]
          tunnel: "Step \ntime \n(ms)" -> [_ w433]
          tunnel: "Step \ntime \n(ms)" -> [w397 _]
          frame False {
            n204 = case shown="True" w399 {
              selector: w399 -> [_ w410]
              tunnel: w403 -> [w406 w417]
              tunnel: w401 -> [w405 _]
              tunnel: w400 -> [w404 w416]
              tunnel: w398 -> [_ w415]
              tunnel: w397 -> [_ w412]
              tunnel: w396 -> [_ w411]
              frame False {
                n205 = case shown="True" w405 {
                  tunnel: w404 -> [_ w408]
                  tunnel: w406 -> [_ w407]
                  frame False {
                  }
                  frame True {
                    n206 = Lossy Enqueue Element(queue=w407, element=w408) -> ()  [unwired: 1 in, 4 out]
                  }
                }
              }
              frame True {
                n207 = property on="stop \nsqueezing" class="Bool"("Visible"=w410) -> ()  [unwired: 2 in, 2 out]
                n208 = while {
                  tunnel: w417 -> [w432]
                  tunnel: w416 -> [w431]
                  tunnel: w415 -> [w430]
                  tunnel: "Outer bound" -> [w429]
                  tunnel: "Inner bound" -> [w428]
                  tunnel: w411 -> [w427]
                  tunnel: [FALSE ("Squeeze")] -> w409
                  tunnel: w412 -> [w420]
                  i -> [w424]
                  stop <- w419 stop-if-true
                  n209 = Equal To 0?(x=w424) -> (x = 0?=w423:bool)
                  n210 = call "Squeeze group (SubVI).vi"("reset"=w423, "Step length"=w427, "Inner bound"=w428, "Outer bound"=w429, "Trap cluster in"=w431, "ROI in"=w430) -> ("output cluster"=w426:T5)  [unwired: 5 in]
                  n211 = Enqueue Element(queue=w432, element=w426, timeout in ms (-1)=1000) -> ()  [unwired: 1 in, 3 out]
                  n212 = Wait (ms)(milliseconds to wait=w420) -> ()  [unwired: 1 out]
                  n213 = local read "Stop program"() -> (w418:bool)
                  n214 = Or(x=w418, y="stop \nsqueezing") -> (x .or. y?=w419:bool)
                }
                n215 = property on="Squeeze" class="Bool (strict)"("Value"=w409) -> ()  [unwired: 2 in, 2 out]
                n216 = property on="stop \nsqueezing" class="Bool"("Visible"=w409) -> ()  [unwired: 2 in, 2 out]
              }
            }
          }
          frame True {
            n217 = Lossy Enqueue Element "Enqueue\noverlay pos"(queue=w439, element=w434) -> ()  [unwired: 1 in, 4 out]
            n218 = case "Add wpt" shown="True" w447 {
              tunnel: w434 -> [_ w528]
              tunnel: w440 -> [w525 w529]
              tunnel: [w525 w526] -> w450
              tunnel: [_ w527] -> w442
              frame False {
              }
              frame True {
                n219 = Enqueue Element "Enqueue path\n waypts"(queue=w529, element=w528) -> (queue out=w526:refnum<queue>, error out=w527:errorcluster)  [unwired: 2 in, 1 out]
              }
            }
            n220 = case "Compute path" shown="True" w446 {
              tunnel: w450 -> [_ w536]
              tunnel: w444 -> [_ w535]
              tunnel: w449 -> [_ w534]
              tunnel: w448 -> [_ w533]
              tunnel: [w530 w531] -> w443
              tunnel: w442 -> [w530 w532]
              frame False {
              }
              frame True {
                n221 = call "compute path cluster.vi"("path queue"=w535, "Arrive simultaeously"=w533, "error in (no error)"=w532, "Step length\n(IMAQ pixels)"=w534, "waypoint queue"=w536) -> ("error out"=w531:errorcluster)  [unwired: 2 in]
              }
            }
            n222 = case "Follow path" shown="True" w445 {
              tunnel: w444 -> [_ w480]
              tunnel: w443 -> [_ w481]
              tunnel: w441 -> [_ w483]
              tunnel: w440 -> [_ w482]
              tunnel: w438 -> [_ w479]
              tunnel: w437 -> [w452 w460]
              tunnel: [w452 w459] -> w436
              tunnel: [w451 w454] -> w435
              tunnel: w434 -> [w451 _]
              tunnel: w433 -> [_ w453]
              frame False {
              }
              frame True {
                w474 = TRUE ("Visible")
                n223 = local write "Display path"(FALSE ("Display path")) -> ()
                n224 = Flush Queue "Flush Waypts"(queue=w482, error in (no error)=w481) -> (error out=w473:errorcluster)  [unwired: 2 out]
                n225 = Get Queue Status(queue=w480, error in (no error)=w473) -> (queue out=w477:refnum<queue>, error out=w472:errorcluster, # elements in queue=w476:i32)  [unwired: 1 in, 5 out]
                n226 = property on="Pause" class="Bool (strict)"(error in=w472, "Visible"=w474) -> (error out=w471:errorcluster)  [unwired: 1 in, 1 out]
                n227 = property on="cancel path" class="Bool"(error in=w471, "Visible"=w474) -> (error out=w470:errorcluster)  [unwired: 1 in, 1 out]
                n228 = for {
                  N: w476 -> [_]
                  tunnel: w470 -> [w503]
                  tunnel: w483 -> [w505]
                  tunnel: w477 -> [w501]
                  tunnel: [w501] -> w475
                  tunnel: [FALSE ("Group traps")] -> w455
                  shift-right: [w492] -> w454
                  shift-left: _ -> [w494]
                  tunnel: [w491] -> w469
                  tunnel: [w488] -> w467 mode=indexing
                  tunnel: [w489] -> w463
                  tunnel: [TRUE ("Display path")] -> w461
                  tunnel: w453 -> [w484]
                  i -> [w489]
                  stop <- w498 stop-if-true
                  n229 = Dequeue Element(queue=w501, timeout in ms (-1)=0, error in (no error)=w503) -> (element=w493:T5, timed out?=w497:bool, error out=w504:errorcluster)  [unwired: 1 out]
                  n230 = while {
                    tunnel: [w522] -> w495
                    tunnel: ["cancel path"] -> w490
                    tunnel: w484 -> [w519]
                    stop <- w524 stop-if-true
                    n231 = local read "Stop program"() -> (w522:bool)
                    n232 = Wait (ms)(milliseconds to wait=w519) -> ()  [unwired: 1 out]
                    n233 = Or(x=w522, y="cancel path") -> (x .or. y?=w520:bool)
                    n234 = Implies(1:w520, 2:"Pause") -> (0:w524:bool)
                  }
                  n235 = case shown="True" "Skip step if \ntimed out" {
                    tunnel: w505 -> [w511 w516]
                    tunnel: w504 -> [w510 w514]
                    tunnel: [FALSE ("overflow?") w512] -> w496
                    tunnel: w493 -> [w509 w515]
                    tunnel: [w508 w513] -> w491
                    tunnel: 500 ("timeout in ms (-1)") -> [w507 _]
                    frame False {
                      n236 = Enqueue Element "Enqueue trap pos"(queue=w511, element=w509, timeout in ms (-1)=w507, error in (no error)=w510) -> (error out=w508:errorcluster)  [unwired: 2 out]
                    }
                    frame True {
                      n237 = Lossy Enqueue Element(queue=w516, element=w515, error in (no error)=w514) -> (overflow?=w512:bool, error out=w513:errorcluster)  [unwired: 2 out]
                    }
                  }
                  "Step \nskipped" <- w496
                  n238 = case shown="False" w495 {
                    tunnel: w494 -> [_ w518]
                    tunnel: w493 -> [w517 _]
                    tunnel: [w517 w518] -> w492
                    frame False {
                    }
                    frame True {
                    }
                  }
                  n239 = Or(x=w490, y=w495) -> (x .or. y?=w500:bool)
                  n240 = Or(x=w500, y=w497) -> (x .or. y?=w498:bool)
                  n241 = Tick Count (ms)() -> (millisecond timer value=w488:u32)
                }
                n242 = local read "Transpose SLM"() -> (w457:bool)
                n243 = call "Trap cluster 2 ROI.vi"("Switch X/Y"=w457, "Trap cluster"=w454, "ROI in"=w479) -> ("ROI out"=w478:T2)
                n244 = local write "Step \nskipped"(w455) -> ()
                n245 = local write "Create path"(w455) -> ()
                n246 = local write "Display path"(w461) -> ()
                n247 = local write "Group \nTraps"(w455) -> ()
                n248 = property on="Pause" class="Bool (strict)"(error in=w469, "Visible"=w455, "Value"=w455) -> (error out=w468:errorcluster)  [unwired: 1 in, 1 out]
                n249 = property on="cancel path" class="Bool"(error in=w468, "Visible"=w455) -> ()  [unwired: 1 in, 2 out]
                n250 = property on="follow path" class="Bool (strict)"("Value"=w455) -> ()  [unwired: 2 in, 2 out]
                n251 = property on="Monitor image" class="ImageControl"(error in=w460, "ROI"=w478) -> (error out=w459:errorcluster)  [unwired: 1 in, 1 out]
                n252 = Array Max & Min(array=w467) -> (max value=w466:u32, min value=w465:u32)  [unwired: 2 out]
                n253 = Subtract(x=w466, y=w465) -> (x-y=w464:u32)
                n254 = Increment(x=w463) -> (x+1=w458:i32)
                n255 = Divide(x=w464, y=w458) -> (x/y=→"Average step \ntime (ms)":dbl)
                n256 = Flush Queue "Flush Path"(queue=w475) -> ()  [unwired: 1 in, 3 out]
              }
            }
          }
        }
        n257 = First Call?() -> (First Call?: T/F=w297:bool)
        n258 = Or(x="Apply Corrections", y=w297) -> (x .or. y?=w298:bool)
        n259 = case shown="True" w298 {
          frame False {
          }
          frame True {
            n260 = call "Apply Corrections.vi"() -> ()  [unwired: 1 in]
          }
        }
      }
      frame True {
        n261 = property on="Cancel calibration" class="Bool"("Visible"=w539) -> ()  [unwired: 2 in, 2 out]
        n262 = flat-sequence {
          tunnel: [w564] -> w551
          tunnel: [w566] -> w550
          tunnel: w546 -> [w564]
          tunnel: [w556] -> w545
          tunnel: [w553] -> w544
          tunnel: w543 -> [w558]
          tunnel: [w557] -> w541
          tunnel: [w629] -> w549
          tunnel: w551 -> [w629]
          tunnel: w550 -> [w587]
          tunnel: [w625] -> w548
          tunnel: w547 -> [w628]
          tunnel: w545 -> [w627]
          tunnel: w544 -> [w624]
          tunnel: [w623] -> w542
          tunnel: w541 -> [w623]
          tunnel: [w585] -> w537
          tunnel: w549 -> [w694]
          tunnel: w542 -> [w692]
          tunnel: [w691] -> w540
          frame #0 {
            w567 = u32 8 items=["Zoom Tool"=8, "Selection Tool"=0, "Pan Tool"=9, "Point Tool"=1, "Line Tool"=2, "Rectangle Tool"=3, "Rotated Rectangle Tool"=12, "Polyline Tool"=10, "Polygon Tool"=5, "Freehand Tool"=11, "Closed Freehand Tool"=6, "Ellipse Tool"=4, "Annulus Tool"=7] ("Current ROI Tool")
            n263 = local read "Using monitoring camera\nfor measurements"() -> (w552:bool)
            n264 = local read "Coordinate mapping \n(IMAQ to SLM)"() -> (w553:T3)
            n265 = Bundle By Name(cluster=w553, "sX"=0.0, "sY"=0.0, "cX"=1.0 ("sX"), "cY"=1.0) -> (w556:T3)
            n266 = case shown="False" w552 {
              frame False {
                n267 = call <vilib>:"Application Directory.vi"() -> ("Application Directory"=w570:path)
                n268 = Build Path(base path=w570, name or relative path="Sub VIs\\Display Image.vi") -> (appended path=w573:path)
                n269 = Open VI Reference(vi path=w573) -> (vi reference=w572:refnum<vi>)  [unwired: 5 in, 1 out]
                n270 = property class="VI"(reference=w572, "Front Panel.Open"=TRUE ("Front Panel Window:Open")) -> ()  [unwired: 1 in, 2 out]
              }
              frame True {
              }
            }
            n271 = local write "Coordinate mapping \n(IMAQ to SLM)"(w556) -> ()
            n272 = property on="ok" class="Bool"("Visible"=TRUE ("ROI Tool Buttons Visibile:Zoom Tool Button Visible")) -> ()  [unwired: 2 in, 2 out]
            n273 = property on="Monitor image" class="ImageControl"("Current ROI Tool"=w567) -> ()  [unwired: 2 in, 2 out]
            n274 = call <vilib>:"Three Button Dialog.vi"("Center Button Text (\"No\")"="Manual" ("T button name (\"OK\")"), "Left Button Text (\"Yes\")"="Auto" ("F button name (\"Cancel\")"), "message"="Mark the center of the \ndisplayed spot using the \nzoom and the point tool, \nthen click the OK button. \n(Will be repeated three times)") -> ("Which Button?"=w566:T14)  [unwired: 8 in]
            n275 = property on="Monitor image" class="ImageControl"(error in=w558, "ROI"=T2 {"Global Rectangle"=[100, 100, 394, 354], "Contours"=[{"Contour Type"=0, "ROI Type"=1, "Points"=[100, 100]}]} ("ROI 2")) -> (error out=w557:errorcluster)  [unwired: 1 in, 1 out]
          }
          frame #1 {
            w581 = sgl 0.0 ("sX")
            w582 = sgl 1.0 ("cX")
            n276 = local read "Coordinate mapping \n(Monitor to Measurement)"() -> (w574:T3)
            n277 = for {
              tunnel: [w650] -> w618 mode=indexing
              tunnel: [w649] -> w617 mode=indexing
              tunnel: T5[] [{"X (IMAQ)"=[-85.0], "Y (IMAQ)"=[-85.0], "Z"=[0.0], "I"=[100.0], "Trap number"=[0], "ROI number"=[0], "Number of traps"=1, "Group"=[]}, {"X (IMAQ)"=[85.0], "Y (IMAQ)"=[-85.0], "Z"=[0.0], "I"=[100.0], "Trap number"=[0], "ROI number"=[0], "Number of traps"=1, "Group"=[]}, {"X (IMAQ)"=[-85.0], "Y (IMAQ)"=[85.0], "Z"=[0.0], "I"=[100.0], "Trap number"=[0], "ROI number"=[0], "Number of traps"=0, "Group"=[]}] -> [w648] mode=indexing
              tunnel: [w645] -> w605 mode=indexing
              tunnel: [w643] -> w604 mode=indexing
              tunnel: w628 -> [w647]
              tunnel: [w642] -> w593 mode=indexing
              tunnel: [w641] -> w592 mode=indexing
              tunnel: w587 -> [w640]
              tunnel: [w638] -> w586
              stop <- w639 stop-if-true
              n278 = Enqueue Element "Enqueue trap pos"(queue=w647, element=w648) -> ()  [unwired: 2 in, 3 out]
              n279 = case shown="\"Left Button\", Default" w640 {
                tunnel: [w655 w672 _ _] -> w650
                tunnel: [w654 w671 _ _] -> w649
                tunnel: [w651 w669 w682 w683] -> w639
                tunnel: [w653 w666 _ _] -> w642
                tunnel: [w652 w665 _ _] -> w641
                tunnel: [w651 w664 w682 w683] -> w638
                frame "Left Button", Default {
                  n280 = flat-sequence {
                    tunnel: [w663] -> w655
                    tunnel: [w662] -> w654
                    tunnel: [w661] -> w653
                    tunnel: [w660] -> w652
                    tunnel: [FALSE] -> w651
                    frame #0 {
                      n281 = Wait (ms)(milliseconds to wait=u32 300) -> ()  [unwired: 1 out]
                    }
                    frame #1 {
                      n282 = local read "Monitoring image"() -> (w659:T1)
                      n283 = local read "Measurement image"() -> (w658:T1)
                      n284 = call "Find spot in image.vi"("Image"=w659) -> ("Y Centroid"=w662:dbl, "X Centroid"=w663:dbl)  [unwired: 7 in]
                      n285 = call "Find spot in image.vi"("Image"=w658) -> ("Y Centroid"=w660:dbl, "X Centroid"=w661:dbl)  [unwired: 7 in]
                    }
                  }
                }
                frame "Center Button" {
                  n286 = while {
                    tunnel: [w680] -> w670
                    tunnel: [w677] -> w669
                    tunnel: [w675] -> w668
                    tunnel: [w674] -> w664
                    stop <- w678 stop-if-true
                    n287 = local read "Stop program"() -> (w674:bool)
                    n288 = global read "Global variables.vi" "Measurement ROI"() -> (w675:T15)
                    n289 = Wait (ms)(milliseconds to wait=u32 50) -> ()  [unwired: 1 out]
                    n290 = Or(x=w674, y="Cancel calibration") -> (x .or. y?=w677:bool)
                    n291 = property on="Monitor image" class="ImageControl"() -> ("ROI"=w680:T2)  [unwired: 2 in, 2 out]
                    n292 = Or(x="ok", y=w677) -> (x .or. y?=w678:bool)
                  }
                  n293 = Unbundle By Name(w668) -> ("Global Rectangle"=w667:i32[])  [unwired: 1 out]
                  n294 = Unbundle By Name(w670) -> ("Global Rectangle"=w673:i32[])  [unwired: 1 out]
                  n295 = Index Array(array=w673) -> (element #1=w672:i32, element #2=w671:i32)  [unwired: 2 in]
                  n296 = Index Array(array=w667) -> (element #1=w666:i32, element #2=w665:i32)  [unwired: 2 in]
                }
                frame "Right Button" {
                  w682 = TRUE
                }
                frame "Window Close" {
                  w683 = TRUE
                }
              }
              n297 = Unbundle By Name(w648) -> ("X (IMAQ)"=w646:sgl[], "Y (IMAQ)"=w644:sgl[])
              n298 = Index Array(array=w644) -> (element=w643:sgl)  [unwired: 1 in]
              n299 = Index Array(array=w646) -> (element=w645:sgl)  [unwired: 1 in]
            }
            n300 = Index Array(array=w617) -> (element #1=w619:dbl, element #2=w620:dbl)  [unwired: 2 in]
            n301 = Index Array(array=w618) -> (element #1=w621:dbl, element #2=w622:dbl)  [unwired: 2 in]
            n302 = Subtract(x=w622, y=w621) -> (x-y=w614:dbl)
            n303 = Subtract(x=w620, y=w619) -> (x-y=w612:dbl)
            n304 = Absolute Value(x=w612) -> (abs(x)=w611:dbl)
            n305 = Absolute Value(x=w614) -> (abs(x)=w613:dbl)
            n306 = Less?(x=w613, y=w611) -> (x < y?=w577:bool)
            n307 = case shown="False" w577 {
              tunnel: w618 -> [w635 w637]
              tunnel: w617 -> [w634 w636]
              tunnel: [w634 w637] -> w615
              tunnel: [w635 w636] -> w616
              frame False {
              }
              frame True {
              }
            }
            n308 = Index Array(array=w592) -> (element #1=w597:dbl, element #2=w596:dbl)  [unwired: 2 in]
            n309 = Index Array(array=w593) -> (element #1=w595:dbl, element #2=w594:dbl)  [unwired: 2 in]
            n310 = Subtract(x=w594, y=w595) -> (x-y=w598:dbl)
            n311 = Subtract(x=w596, y=w597) -> (x-y=w600:dbl)
            n312 = Absolute Value(x=w600) -> (abs(x)=w601:dbl)
            n313 = Absolute Value(x=w598) -> (abs(x)=w599:dbl)
            n314 = Less?(x=w599, y=w601) -> (x < y?=w578:bool)
            n315 = case shown="False" w578 {
              tunnel: w593 -> [w631 w633]
              tunnel: w592 -> [w630 w632]
              tunnel: [w630 w633] -> w602
              tunnel: [w631 w632] -> w603
              frame False {
              }
              frame True {
              }
            }
            n316 = formula code="cX = (xSLM[1] - xSLM[0]) / (xMonitor[1] - xMonitor[0]); \ncY = (ySLM[2] - ySLM[0]) / (yMonitor[2] - yMonitor[0]); \n\nsX = xSLM[0] - xMonitor[0] *cX;\nsY = ySLM[0] - yMonitor[0] *cY;\n\ncXm = (xMeasure[1] - xMeasure[0]) / (xMonitor[1] - xMonitor[0]); \ncYm = (yMeasure[2] - yMeasure[0]) / (yMonitor[2] - yMonitor[0]); \n\nsXm = xMeasure[0] - xMonitor[0] *cXm;\nsYm = yMeasure[0] - yMonitor[0] *cYm;"("xMonitor"=w616, "yMonitor"=w615, "xSLM"=w605, "ySLM"=w604, "xMeasure"=w603, "yMeasure"=w602) -> ("cX"=w610:dbl, "cY"=w609:dbl, "sX"=w608:dbl, "sY"=w607:dbl, "cXm"=w591:dbl, "cYm"=w590:dbl, "sXm"=w589:dbl, "sYm"=w588:dbl)
            n317 = local read "Using monitoring camera\nfor measurements"() -> (w576:bool)
            n318 = Select(t=FALSE, s=w576, f=w578) -> (s? t:f=w579:bool)
            n319 = Bundle By Name(cluster=w627, "cX"=w610, "cY"=w609, "sX"=w608, "sY"=w607) -> (w626:T3)
            n320 = Bundle By Name(cluster=w574, "cX"=w582, "cY"=w582, "sX"=w581, "sY"=w581) -> (w580:T3)
            n321 = Bundle By Name(cluster=w574, "cX"=w591, "cY"=w590, "sX"=w589, "sY"=w588) -> (w583:T3)
            n322 = Select(t=w580, s=w576, f=w583) -> (s? t:f=w584:T3)
            n323 = case "Calibration canceled?" shown="True" w586 {
              tunnel: w626 -> [w687 _]
              tunnel: [w687 w689] -> w625
              tunnel: w624 -> [_ w689]
              tunnel: [w684 w688] -> w585
              tunnel: w584 -> [w684 _]
              tunnel: w579 -> [w686 _]
              tunnel: w577 -> [w685 _]
              tunnel: w574 -> [_ w688]
              frame False {
                n324 = local write "Transpose Measurement"(w686) -> ()
                n325 = local write "Transpose SLM"(w685) -> ()
              }
              frame True {
              }
            }
          }
          frame #2 {
            w690 = FALSE ("ROI Tool Buttons Visibile:Zoom Tool Button Visible")
            w693 = u32 1 items=["Zoom Tool"=8, "Selection Tool"=0, "Pan Tool"=9, "Point Tool"=1, "Line Tool"=2, "Rectangle Tool"=3, "Rotated Rectangle Tool"=12, "Polyline Tool"=10, "Polygon Tool"=5, "Freehand Tool"=11, "Closed Freehand Tool"=6, "Ellipse Tool"=4, "Annulus Tool"=7] ("Current ROI Tool")
            n326 = property on="Monitor image" class="ImageControl"(error in=w692, "ROI"=w694) -> (error out=w691:errorcluster)  [unwired: 1 in, 1 out]
            n327 = property on="Monitor image" class="ImageControl"("Current ROI Tool"=w693, "Point Tool Button Visibile"=w690) -> ()  [unwired: 2 in, 2 out]
            n328 = property on="Cancel" class="Bool"("Visible"=w690) -> ()  [unwired: 2 in, 2 out]
            n329 = property on="ok" class="Bool"("Visible"=w690) -> ()  [unwired: 2 in, 2 out]
          }
        }
        n330 = local write "Coordinate mapping \n(IMAQ to SLM)"(w548) -> ()
        n331 = local write "Coordinate mapping \n(Monitor to Measurement)"(w537) -> ()
      }
    }
  }
  n332 = while "Hologram generation loop" {
    tunnel: w52 -> [w706]
    tunnel: w30 -> [w704]
    tunnel: w53 -> [w703]
    tunnel: [w702] -> w50
    shift-right: [w701] -> _
    shift-left: _ -> [w700]
    shift-right: [w699] -> _
    shift-left: _ -> [w698]
    shift-right: [w697] -> _
    shift-left: FALSE ("Display hologram\nand computed \nimage plane") -> [w696]
    stop <- w707 stop-if-true
    n333 = Dequeue Element "Dequeue Current \ntrap cluster"(queue=w706, timeout in ms (-1)=1000) -> (element=w705:T5, timed out?=w695:bool)  [unwired: 1 in, 2 out]
    n334 = case shown="False" w695 {
      tunnel: w700 -> [w714 _]
      tunnel: w705 -> [w718 _]
      tunnel: w704 -> [w717 _]
      tunnel: w703 -> [w716 w731]
      tunnel: [w715 w731] -> w702
      tunnel: [w714 "Coordinate mapping \n(IMAQ to SLM)"] -> w701
      tunnel: [w711 "Hologram generation"] -> w699
      tunnel: w698 -> [w711 _]
      tunnel: [w710 "Display hologram\nand computed \nimage plane"] -> w697
      tunnel: w696 -> [w710 _]
      frame False {
        n335 = Unbundle By Name(w711) -> ("Method"=w713:i32, "Iterations"=w712:i32)
        n336 = call "Shift coordinates (IMAQ to SLM).vi"("Trap cluster"=w718, "Coordinate mapping \n(IMAQ to SLM)"=w714) -> ("X (SLM)"=w719:sgl[], "Y (SLM)"=w722:sgl[], "Intensities"=w720:sgl[], "Z (SLM)"=w721:sgl[])  [unwired: 1 in, 1 out]
        n337 = call "Generate Hologram.vi"("x"=w719, "y"=w722, "z"=w721, "spot_intensities"=w720, "CUDA/SLM error in"=w716, "N_iterations"=w712, "method"=w713) -> ("CGH out"=w723:u8[][], "CUDA/SLM error out"=w715:errorcluster)  [unwired: 17 in, 2 out]
        n338 = case "Display current CGH and trap positions.\nCompute and display farfield of current CGH" shown="True" w710 {
          tunnel: w723 -> [_ w727]
          tunnel: w718 -> [w724 w725]
          tunnel: [w724 w725] -> w709
          frame False {
          }
          frame True {
            n339 = call "Calculate farfield intensity.vi"("h_pSLM"=w727, "SLMsize"=512 ("Numeric")) -> ()  [unwired: 1 out]
            "Current trap pos" <- w725
          }
        }
        n340 = Lossy Enqueue Element "Put current trap \ncluster in overlay \nqueue"(queue=w717, element=w709) -> ()  [unwired: 1 in, 4 out]
      }
      frame True {
      }
    }
    n341 = local read "Stop program"() -> (w707:bool)
  }
  n342 = while {
    tunnel: w42 -> [w749]
    tunnel: [w747] -> w35
    tunnel: w34 -> [w748]
    tunnel: w33 -> [w745]
    tunnel: w31 -> [w744]
    tunnel: w30 -> [w743]
    tunnel: w29 -> [w737]
    tunnel: w28 -> [w732]
    stop <- w750 stop-if-true
    n343 = Preview Queue Element(queue=w743, timeout in ms (-1)=10) -> (element=w742:T5)  [unwired: 1 in, 3 out]
    n344 = case shown="False" w745 {
      tunnel: w749 -> [w755 w758]
      tunnel: w748 -> [w754 _]
      tunnel: [w753 w759] -> w741
      tunnel: [w752 w756] -> w747
      tunnel: w744 -> [_ w761]
      frame False {
        n345 = call "Acquire image (SubVI).vi"("Camera type"=w754, "Measurement camera \ncluster in"=w755) -> ("Image Out"=w753:T1, "Measurement camera cluster out"=w752:T10)  [unwired: 7 in, 1 out]
      }
      frame True {
        n346 = Unbundle By Name(w758) -> ("Image"=w762:T1, "Camera error"=w760:errorcluster)
        n347 = call "IMAQ Copy"("error in (no error)"=w760, "Image Dst"=w761, "Image Src"=w762) -> ("error out"=w757:errorcluster, "Image Dst Out"=w759:T1)  [unwired: 3 in]
        n348 = Bundle By Name(cluster=w758, "Camera error"=w757) -> (w756:T10)
      }
    }
    n349 = Wait (ms)(milliseconds to wait=u32 200) -> ()  [unwired: 1 out]
    n350 = local read "Stop program"() -> (w750:bool)
    n351 = local read "ROI \nsize"() -> (w740:dbl)
    n352 = Get Queue Status(queue=w737, return elements? (F)="Display path") -> (elements=w738:T5[])  [unwired: 1 in, 7 out]
    n353 = local read "Transpose SLM"() -> (w739:bool)
    n354 = case shown="True" "Display ROIs" {
      tunnel: w732 -> [_ w751]
      frame False {
      }
      frame True {
        n355 = call "Display ROIs.vi"("ROI array in"=w751) -> ()  [unwired: 11 in]
      }
    }
    n356 = call "Create trap overlay.vi"("Current trap cluster"=w742, "Image in"=w741, "ROI size"=w740, "Switch X/Y"=w739, "Path"=w738) -> ("Image Out"=→"Monitor image":T1)
  }
  n357 = while "Measurement loop" {
    tunnel: w28 -> [w770]
    tunnel: w5 -> [w802]
    shift-right: [w801] -> _
    shift-left: _ -> [w766]
    tunnel: w16 -> [w800]
    shift-right: [w799] -> _
    shift-left: _ -> [w765]
    tunnel: [w776] -> _
    tunnel: w15 -> [w794]
    tunnel: w30 -> [w796]
    tunnel: w29 -> [_]
    tunnel: [w797] -> w45
    tunnel: w13 -> [w784]
    tunnel: w27 -> [w773]
    shift-right: [w795] -> _
    shift-left: w23 -> [w768]
    shift-right: [w790] -> _
    shift-left: _ -> [w767]
    tunnel: w19 -> [w789]
    tunnel: w19 -> [w763]
    tunnel: w17 -> [_]
    tunnel: w14 -> [w782]
    i -> [w792]
    stop <- w803 stop-if-true
    n358 = Or(x=w782, y="Record") -> (x .or. y?=w783:bool)
    n359 = feedback #2() -> (w786:u32)  [unwired: 1 in]
    n360 = case shown="True" w783 {
      tunnel: w794 -> [w827 _]
      tunnel: [w825 w828] -> w793
      tunnel: w792 -> [_ _]
      tunnel: w786 -> [_ w829]
      frame False {
        n361 = Unbundle By Name(w827) -> ("IMAQ Session"=w826:refnum<k11>)
        n362 = call <vilib>:"IMAQ Status.vi"("IMAQ Session In"=w826) -> ("Last Valid Buffer Number"=w825:i32)  [unwired: 6 in, 4 out]
      }
      frame True {
        n363 = Increment(x=w829) -> (x+1=w828:u32)
      }
    }
    n364 = call "Acquire image (SubVI).vi"("Buffer number"=w793, "Camera type"=w784, "Measurement camera \ncluster in"=w794) -> ("Image Out"=w785:T1, "Measurement camera cluster out"=w772:T10, "Buffer Number Out"=w777:u32)  [unwired: 6 in]
    n365 = feedback-in #2(w777) -> ()
    n366 = case shown="True" TRUE {
      tunnel: w777 -> [_ w824]
      frame False {
      }
      frame True {
        n367 = call "IMAQCalculateFPS.vi"("Update interval"=u32 1000, "buffer number"=w824) -> ("processed FPS"=→"processed FPS":dbl, "acquired FPS"=→"acquired FPS":dbl)
      }
    }
    n368 = case shown="True" "subtract\nbackground" {
      tunnel: [w816 w820] -> w788
      tunnel: w785 -> [w816 w819]
      tunnel: w763 -> [_ w817]
      tunnel: [_ w818] -> w780
      tunnel: w773 -> [_ _]
      frame False {
      }
      frame True {
        n369 = call "IMAQ Subtract"("Image Src A"=w819, "Image Src B"=w817) -> ("Image Dst Out"=w820:T1, "error out"=w818:errorcluster)  [unwired: 5 in]
      }
    }
    n370 = case shown="True" "save image" {
      tunnel: w788 -> [w830 w835]
      tunnel: [w830 w834] -> w776
      tunnel: w780 -> [_ _]
      frame False {
      }
      frame True {
        n371 = call "File Dialog"("start path"="Save image path") -> ("selected path"=w833:path, "cancelled"=w832:bool)  [unwired: 11 in, 2 out]
        n372 = case shown="False" w832 {
          tunnel: w835 -> [w838 w839]
          tunnel: [w837 w839] -> w834
          tunnel: w833 -> [w836 _]
          frame False {
            n373 = call-poly "IMAQ Write File 2"("File Path"=w836, "Image"=w838) -> ("Image Out (duplicate)"=w837:T1)  [unwired: 8 in, 1 out]
          }
          frame True {
          }
        }
      }
    }
    n374 = Preview Queue Element(queue=w796) -> (element=w769:T5)  [unwired: 2 in, 3 out]
    n375 = case shown="True" "Calibrate \ntraps" {
      tunnel: w772 -> [w804 w815]
      tunnel: [w804 w815] -> w771
      tunnel: w770 -> [_ w814]
      tunnel: w769 -> [_ w813]
      tunnel: w768 -> [_ w812]
      tunnel: w767 -> [_ w811]
      tunnel: w766 -> [_ w810]
      tunnel: w765 -> [_ w809]
      tunnel: w763 -> [_ w807]
      frame False {
      }
      frame True {
        n376 = call "Acquire calibration sequence (SubVI).vi"("Refnum in"=w807, "output cluster in"=w813, "Calibration \nruns"="Calibration \nruns", "Calibration framerate"="Calibration framerate", "Measurement camera cluster in"=w815, "Measure \nintensities"=w809, "Transpose Measurement"=w811, "N samples"="N samples", "ROI \nsize"=w810, "Array"=w814, "Coordinate mapping \n(Monitor to Measurement)"=w812) -> ()  [unwired: 4 in, 1 out]
      }
    }
    n377 = call "Position measurement.vi"("Measure \nintensities"=w765, "ROI size"=w766, "Acquired Buffer Number"=w786, "Switch xy"=w767, "Coordinate mapping \n(Monitor to Measurement)"=w768, "ROIs"=w770, "Target positions (monitor)"=w769, "Image"=w776) -> ("Target coordinates (measurement)"=w774:cluster{"X target":sgl[], "Y target":sgl[]}, "Position data out (measurement)"=w775:T7)  [unwired: 1 in]
    n378 = feedback #3() -> (w778:u32[])  [unwired: 1 in]
    n379 = case shown="False" "Record" {
      tunnel: w802 -> [w841 w926]
      tunnel: [w841 w925] -> _
      tunnel: [_ w924] -> _
      tunnel: ["ROI \nsize" w923] -> w801
      tunnel: w766 -> [_ w923]
      tunnel: w800 -> [w871 w922]
      tunnel: [w871 w921] -> _
      tunnel: ["Measure \nintensities" w920] -> w799
      tunnel: w765 -> [_ w920]
      tunnel: [FALSE ("timed out?") w918] -> _
      tunnel: w776 -> [w855 _]
      tunnel: w771 -> [w851 w917]
      tunnel: [w865 w917] -> w797
      tunnel: w775 -> [w842 w916]
      tunnel: ["Coordinate mapping \n(Monitor to Measurement)" w915] -> w795
      tunnel: w768 -> [_ w915]
      tunnel: [w859 _] -> _
      tunnel: [w857 w914] -> w790
      tunnel: w767 -> [_ w914]
      tunnel: w789 -> [w854 _]
      tunnel: w785 -> [w852 _]
      tunnel: [w847 w913] -> w779
      tunnel: w778 -> [w848 w911]
      tunnel: w776 -> [w845 _]
      tunnel: w774 -> [w844 w910]
      frame False {
        n380 = Unbundle By Name(w851) -> ("Camera error"=w850:errorcluster)
        n381 = Unbundle By Name(w851) -> ("Camera type"=w853:T8, "Image"=w858:T1)
        n382 = call "IMAQ Quantify 2"("error in (no error)"=w850, "Image"=w852) -> ("error out"=w866:errorcluster, "Global Report"=w864:T4)  [unwired: 7 in, 1 out]
        "Measurement image report" <- w864
        n383 = case shown="True" "Display data" {
          tunnel: w842 -> [_ w873]
          tunnel: w844 -> [_ w872]
          frame False {
          }
          frame True {
            n384 = call "Display Cetroids (SubVI).vi"("Target coordinates"=w872, "Measurement data"=w873) -> ()  [unwired: 7 in, 3 out]
          }
        }
        n385 = Wait (ms)(milliseconds to wait=u32 20) -> ()  [unwired: 1 out]
        n386 = Get Queue Status(queue=w841) -> (# elements in queue=→"# recorded points":i32)  [unwired: 2 in, 7 out]
        n387 = case shown="\"IMAQ ring\"" w853 {
          tunnel: w855 -> [_ w909]
          tunnel: w858 -> [_ w908]
          frame "IMAQ (Camera Link)", Default {
          }
          frame "IMAQ ring" {
            n388 = call "IMAQ Copy"("Image Dst"=w908, "Image Src"=w909) -> ("error out"=w907:errorcluster)  [unwired: 4 in, 1 out]
            n389 = call <vilib>:"Clear Errors.vi"("error in (no error)"=w907) -> ()  [unwired: 6 in, 1 out]
          }
        }
        n390 = Unbundle By Name(w864) -> ("Maximal Value"=w863:sgl)
        n391 = Bundle By Name(cluster=w851, "Camera error"=w866) -> (w865:T10)
        n392 = case shown="True" "Display meas image" {
          tunnel: w845 -> [_ w874]
          frame False {
          }
          frame True {
            n393 = call "Display Image.vi"("Image 2"=w874) -> ()  [unwired: 11 in]
          }
        }
        n394 = case shown="False" "store \nbackground" {
          tunnel: w854 -> [w894 w905]
          tunnel: w851 -> [_ w904]
          tunnel: w853 -> [_ w903]
          frame False {
            n395 = Not(x="Increment") -> (.not. x?=w888:bool)
            n396 = And(x="decrement", y=w888) -> (x .and. y?=w890:bool)
            n397 = case shown="True" "Increment" {
              tunnel: w894 -> [_ w900]
              tunnel: [sgl 0.0 ("Constant") w899] -> w893
              frame False {
              }
              frame True {
                w899 = sgl 1.0 ("Constant")
                n398 = call "IMAQ Add"("Image Src A"=w900, "Constant"=w899) -> ()  [unwired: 5 in, 2 out]
              }
            }
            n399 = case shown="True" w890 {
              tunnel: w894 -> [_ w897]
              tunnel: w893 -> [w895 _]
              tunnel: [w895 w896] -> w892
              frame False {
              }
              frame True {
                w896 = sgl -1.0 ("Constant")
                n400 = call "IMAQ Add"("Image Src A"=w897, "Constant"=w896) -> ()  [unwired: 5 in, 2 out]
              }
            }
            n401 = feedback #4(sgl 0.0) -> (w886:sgl)
            "threshold" <- w886
            n402 = Add(x=w892, y=w886) -> (x+y=w887:sgl)
            n403 = feedback-in #4(w887) -> ()
          }
          frame True {
            n404 = call "Acquire average image (SubVI).vi"("Camera type"=w903, "Measurement camera cluster in"=w904, "averaging time (ms)"=1000) -> ("Refnum out"=w901:T1)  [unwired: 8 in]
            n405 = call "IMAQ Copy"("Image Dst"=w905, "Image Src"=w901) -> ("error out"=w906:errorcluster)  [unwired: 4 in, 1 out]
            n406 = call <vilib>:"Clear Errors.vi"("error in (no error)"=w906) -> ()  [unwired: 6 in, 1 out]
          }
        }
        n407 = Greater Or Equal?(x=w863, y=sgl 210.0) -> (x >= y?=→"Image\nsaturated":bool)
        n408 = local read "Using monitoring camera\nfor measurements"() -> (w859:bool)
        n409 = case shown="True" "reset" {
          tunnel: w848 -> [w875 w881]
          tunnel: [w875 u32[] [] ("t")] -> w847
          frame False {
          }
          frame True {
            n410 = Array Max & Min(array=w881) -> (max value=w883:u32, min value=w882:u32)  [unwired: 2 out]
            n411 = Subtract(x=w883, y=w882) -> (x-y=w879:u32)
            n412 = Array Size(array=w881) -> (size(s)=w880:i32)
            n413 = Decrement(x=w880) -> (x-1=w878:i32)
            n414 = Divide(x=w878, y=w879) -> (x/y=w877:dbl)
            n415 = Multiply(x=w877, y=1000.0) -> ()  [unwired: 1 out]
          }
        }
        n416 = local read "Transpose Measurement"() -> (w857:bool)
      }
      frame True {
        n417 = Enqueue Element(queue=w922, element=w910) -> (queue out=w921:refnum<queue>)  [unwired: 2 in, 2 out]
        n418 = Enqueue Element(queue=w926, element=w916, timeout in ms (-1)=10000) -> (queue out=w925:refnum<queue>, timed out?=w918:bool, error out=w924:errorcluster)  [unwired: 1 in]
        n419 = Tick Count (ms)() -> (millisecond timer value=w912:u32)
        n420 = Build Array (concatenate)(w911, w912) -> (w913:u32[])
      }
    }
    n421 = feedback-in #3(w779) -> ()
    n422 = local read "Stop program"() -> (w803:bool)
  }
  n423 = Unbundle By Name(w35) -> ("Camera type"=w41:T8, "IMAQ Session"=w40:refnum<k11>, "IMAQdx Session"=w39:T9, "Camera error"=w38:errorcluster, "Image"=w37:T1, "Image buffers"=w36:T1[])
  n424 = call "FreeGPUandSLM.vi"("error in"=w50) -> ("error out"=w69:errorcluster)  [unwired: 1 out]
  "CUDA/SLM error" <- w69
  n425 = property on="ROI \nsize" class="DigNum (strict)"("Visible"=w78) -> ()  [unwired: 2 in, 2 out]
  n426 = property on="Record" class="Bool (strict)"("Visible"=w78) -> ()  [unwired: 2 in, 2 out]
  n427 = property on="Save data" class="Bool"("Visible"=w78) -> ()  [unwired: 2 in, 2 out]
  n428 = property on="Measure \nintensities" class="Bool (strict)"("Visible"=w78) -> ()  [unwired: 2 in, 2 out]
  n429 = property on="Purge data" class="Bool"("Visible"=w78) -> ()  [unwired: 2 in, 2 out]
  n430 = case shown="\"IMAQdx (firewire)\"" w41 {
    tunnel: w40 -> [w930 _ _ w938]
    tunnel: [w929 _ w934 w937] -> _
    tunnel: w39 -> [_ w933 _ _]
    tunnel: w38 -> [w928 w932 w934 w936]
    tunnel: w37 -> [w927 w931 _ _]
    tunnel: w36 -> [_ _ _ w935]
    frame "IMAQ (Camera Link)", Default {
      n431 = call <vilib>:"IMAQ Close.vi"("error in (no error)"=w928, "IMAQ Session In"=w930) -> ("error out"=w929:errorcluster)  [unwired: 9 in]
      n432 = call "IMAQ Dispose"("Image"=w927) -> ()  [unwired: 5 in, 1 out]
    }
    frame "IMAQdx (firewire)" {
      n433 = call <vilib>:"IMAQdx Close Camera.vi"("error in"=w932, "Session In"=w933) -> ()  [unwired: 9 in, 1 out]
      n434 = call "IMAQ Dispose"("Image"=w931) -> ()  [unwired: 5 in, 1 out]
    }
    frame "No camera" {
    }
    frame "IMAQ ring" {
      n435 = call <vilib>:"IMAQ Close.vi"("error in (no error)"=w936, "IMAQ Session In"=w938) -> ("error out"=w937:errorcluster)  [unwired: 9 in]
      n436 = for {
        tunnel: w935 -> [w939] mode=indexing
        n437 = call "IMAQ Dispose"("Image"=w939) -> ()  [unwired: 5 in, 1 out]
      }
    }
  }
  n438 = call-poly <vilib>:"Close Input Device.vi"("error in (no error)"=w66, "device ID"=w67) -> ()  [unwired: 9 out]
  n439 = Unbundle By Name(w72) -> ("Contours"=w77:T16)
  n440 = Index Array(array=w77) -> (element=w76:T17)  [unwired: 1 in]
  n441 = flat-sequence {
    tunnel: w69 -> [_]
    tunnel: w68 -> [_]
    frame #0 {
      n442 = local write "Stop program"(FALSE ("Stop program")) -> ()
    }
  }
  n443 = Unbundle By Name(w76) -> ("ROI Type"=w75:u32)
  n444 = Equal?(x=w75, y=u32 1) -> (x = y?=w73:bool)
  n445 = Unbundle By Name(w45) -> ("Camera type"=w49:T8, "IMAQ Session"=w48:refnum<k11>, "IMAQdx Session"=w47:T9, "Camera error"=w46:errorcluster, "Image"=w44:T1, "Image buffers"=w43:T1[])
  n446 = case shown="True" w73 {
    tunnel: w72 -> [_ w941]
    frame False {
    }
    frame True {
      n447 = local write "ROI"(w941) -> ()
    }
  }
  n448 = case shown="\"IMAQ (Camera Link)\", Default" w49 {
    tunnel: w48 -> [w945 _ _ w954]
    tunnel: [w944 w949 w950 w953] -> w71
    tunnel: w47 -> [_ w948 _ _]
    tunnel: w46 -> [w943 w947 w950 w952]
    tunnel: w44 -> [w942 w946 _ _]
    tunnel: w43 -> [_ _ _ w951]
    frame "IMAQ (Camera Link)", Default {
      n449 = call <vilib>:"IMAQ Close.vi"("error in (no error)"=w943, "IMAQ Session In"=w945) -> ("error out"=w944:errorcluster)  [unwired: 9 in]
      n450 = call "IMAQ Dispose"("Image"=w942) -> ()  [unwired: 5 in, 1 out]
    }
    frame "IMAQdx (firewire)" {
      n451 = call <vilib>:"IMAQdx Close Camera.vi"("error in"=w947, "Session In"=w948) -> ("error out"=w949:errorcluster)  [unwired: 9 in]
      n452 = call "IMAQ Dispose"("Image"=w946) -> ()  [unwired: 5 in, 1 out]
    }
    frame "No camera" {
    }
    frame "IMAQ ring" {
      n453 = for {
        tunnel: w951 -> [w955] mode=indexing
        n454 = call "IMAQ Dispose"("Image"=w955) -> ()  [unwired: 5 in, 1 out]
      }
      n455 = call <vilib>:"IMAQ Close.vi"("error in (no error)"=w952, "IMAQ Session In"=w954) -> ("error out"=w953:errorcluster)  [unwired: 9 in]
    }
  }
  n456 = Merge Errors(w71, w70) -> (w68:errorcluster)
  "NI Vision error" <- w68
